vi "Measure vs B2Dv8.vi"() -> ()   [LabVIEW 2009]
doc: "This VI is an example operator panel.\n\nThe VI contains a table for the field values that may be configured manually, or loaded by checking the \"Prompt for File\" box. The data file should contain 3 columns of data, with each column delimited by a tab character.\n\nBefore the VI is executed, set the desired field units and coordinate system. Once the VI is started, follow the directions in the STATUS indicator to operate. Once a field value is achieved, it will be held indefinitely with no user intervention.\n\nThe present field is displayed in the selected units and coordinate system. The present field is queried once per second.\n\nIf a field point is specified that is outside the limits for the magnet, the VI will abort execution."
uses:
  <vilib>/Utility/file.llb/Read From Spreadsheet File (DBL).vi
panel:
  in  "Nr. of Accumulations":i32=5
  out "appended array":dbl[](array[numeric])=[3.4997816518320115, 222.76394903933627, 0.0, 0.0, 0.0, 0.0, 0.0, 0.0, 0.0, 0.0, 26.935568000000004, 3405678871.716173]
  in  "X Axis":enum16{"B", "phi"}(ring)=enum."phi"
  in  "Y Axis":T1(ring)=enum."HP (V)"
  out "XY Graph":T2(graph)
  in  "GPIB HP 2":string="13"
  in  "Wait between \nVectors":bool=TRUE
  in  "Change\nPID\n(polar coordinates)":bool=TRUE
  in  "Wait between \nVectors (ms)":u32=4000
  out "measured data":dbl[][](array[numeric])=[[3.500030260354902, 90.02209961014816, 0.0, 0.0, 0.0, 0.0, 0.0, 0.0, 0.0, 0.0, -94.19115, 3405672865.0000706], [3.5000353306931054, 90.40008745596127, 0.0, 0.0, 0.0, 0.0, 0.0, 0.0, 0.0, 0.0, -93.17439999999999, 3405672888.556781], [3.500010167370946, 90.77498772333144, 0.0, 0.0, 0.0, 0.0, 0.0, 0.0, 0.0, 0.0, -92.12794, 3405672906.302329], [3.499961687061731, 91.1795707814255, 0.0, 0.0, 0.0, 0.0, 0.0, 0.0, 0.0, 0.0, -90.85747400000001, 3405672924.971062], [3.50004724865251, 91.57794022797674, 0.0, 0.0, 0.0, 0.0, 0.0, 0.0, 0.0, 0.0, -88.536796, 3405672943.172702], [3.500004245611711, 91.97742193199196, 0.0, 0.0, 0.0, 0.0, 0.0, 0.0, 0.0, 0.0, -86.630854, 3405672961.1512966], [3.499981515165474, 92.3769958711717, 0.0, 0.0, 0.0, 0.0, 0.0, 0.0, 0.0, 0.0, -84.437106, 3405672979.515969], [3.499989652556133, 92.77683009737729, 0.0, 0.0, 0.0, 0.0, 0.0, 0.0, 0.0, 0.0, -82.45712800000001, 3405672997.6575966], [3.499997929856531, 93.17958494444387, 0.0, 0.0, 0.0, 0.0, 0.0, 0.0, 0.0, 0.0, -80.15669, 3405673015.994263], [3.4999788975649553, 93.57973481313714, 0.0, 0.0, 0.0, 0.0, 0.0, 0.0, 0.0, 0.0, -77.925174, 3405673034.877039], [3.50003012194181, 93.97981982914929, 0.0, 0.0, 0.0, 0.0, 0.0, 0.0, 0.0, 0.0, -75.205726, 3405673052.8976426], [3.4999928001068805, 94.37806425473491, 0.0, 0.0, 0.0, 0.0, 0.0, 0.0, 0.0, 0.0, -72.669112, 3405673070.9132447], [3.5000066802793395, 94.77875900181826, 0.0, 0.0, 0.0, 0.0, 0.0, 0.0, 0.0, 0.0, -69.859166, 3405673089.0468707], [3.499968184726827, 95.17532458941045, 0.0, 0.0, 0.0, 0.0, 0.0, 0.0, 0.0, 0.0, -66.825818, 3405673107.0374684], [3.499973556528678, 95.57470930884492, 0.0, 0.0, 0.0, 0.0, 0.0, 0.0, 0.0, 0.0, -63.7532, 3405673125.491158], [3.4999261373920447, 95.97066938046576, 0.0, 0.0, 0.0, 0.0, 0.0, 0.0, 0.0, 0.0, -60.45445599999999, 3405673143.7017994], [3.5000298004588473, 96.38048701574986, 0.0, 0.0, 0.0, 0.0, 0.0, 0.0, 0.0, 0.0, -57.068999999999996, 3405673162.2455077], [3.500064831970974, 96.77557569619363, 0.0, 0.0, 0.0, 0.0, 0.0, 0.0, 0.0, 0.0, -53.408407999999994, 3405673180.1530886], [3.4999764736352157, 97.1788243385936, 0.0, 0.0, 0.0, 0.0, 0.0, 0.0, 0.0, 0.0, -49.82861199999999, 3405673198.7077985], [3.499899112903114, 97.5720228055998, 0.0, 0.0, 0.0, 0.0, 0.0, 0.0, 0.0, 0.0, -46.072646, 3405673217.375531], [3.4999856331847994, 97.97927285454584, 0.0, 0.0, 0.0, 0.0, 0.0, 0.0, 0.0, 0.0, -42.447092, 3405673235.5991755], [3.4999729959101114, 98.3805293531586, 0.0, 0.0, 0.0, 0.0, 0.0, 0.0, 0.0, 0.0, -38.347238, 3405673254.280911], [3.499991174417444, 98.77649336396482, 0.0, 0.0, 0.0, 0.0, 0.0, 0.0, 0.0, 0.0, -34.288334, 3405673272.973649], [3.5000539345844377, 99.1754114769969, 0.0, 0.0, 0.0, 0.0, 0.0, 0.0, 0.0, 0.0, -30.040484, 3405673291.4163365], [3.5000102512135594, 99.57505833083601, 0.0, 0.0, 0.0, 0.0, 0.0, 0.0, 0.0, 0.0, -25.978331999999998, 3405673309.6199765], [3.5000214011488553, 99.98001455890109, 0.0, 0.0, 0.0, 0.0, 0.0, 0.0, 0.0, 0.0, -21.579306000000003, 3405673327.64058], [3.4999851274255445, 100.3796233603908, 0.0, 0.0, 0.0, 0.0, 0.0, 0.0, 0.0, 0.0, -17.288418, 3405673346.434338], [3.499954446117835, 100.77906761278494, 0.0, 0.0, 0.0, 0.0, 0.0, 0.0, 0.0, 0.0, -12.950921999999998, 3405673365.5421586], [3.4999038351503318, 101.17711177650253, 0.0, 0.0, 0.0, 0.0, 0.0, 0.0, 0.0, 0.0, -8.468328, 3405673383.8398175], [3.5000326492762897, 101.57761950670657, 0.0, 0.0, 0.0, 0.0, 0.0, 0.0, 0.0, 0.0, -4.102902, 3405673402.066462], [3.5000535285620993, 101.98021835524455, 0.0, 0.0, 0.0, 0.0, 0.0, 0.0, 0.0, 0.0, 0.38745399999999997, 3405673420.2901063], [3.4999165652340913, 102.3749303639201, 0.0, 0.0, 0.0, 0.0, 0.0, 0.0, 0.0, 0.0, 4.841813999999999, 3405673438.627773], [3.5000474151074012, 102.77699848468114, 0.0, 0.0, 0.0, 0.0, 0.0, 0.0, 0.0, 0.0, 9.427456000000001, 3405673456.962439], [3.4999308826603994, 103.17911248439914, 0.0, 0.0, 0.0, 0.0, 0.0, 0.0, 0.0, 0.0, 13.765427999999998, 3405673475.7191896], [3.5000704905187265, 103.57366085912142, 0.0, 0.0, 0.0, 0.0, 0.0, 0.0, 0.0, 0.0, 261.09814400000005, 3405673493.5167484], [3.4999923875488643, 103.97478211562277, 0.0, 0.0, 0.0, 0.0, 0.0, 0.0, 0.0, 0.0, 265.36180399999995, 3405673511.973439], [3.50008904903861, 104.37808498401525, 0.0, 0.0, 0.0, 0.0, 0.0, 0.0, 0.0, 0.0, 229.417352, 3405673530.1890817], [3.4999492656037177, 104.77837537502313, 0.0, 0.0, 0.0, 0.0, 0.0, 0.0, 0.0, 0.0, 232.49712, 3405673548.7317896], [3.50001056744119, 105.17362498473213, 0.0, 0.0, 0.0, 0.0, 0.0, 0.0, 0.0, 0.0, 235.83822400000003, 3405673567.045451], [3.5000558796967804, 105.57885121352332, 0.0, 0.0, 0.0, 0.0, 0.0, 0.0, 0.0, 0.0, 239.56730199999998, 3405673585.022046], [3.5000177358693487, 105.97640425681314, 0.0, 0.0, 0.0, 0.0, 0.0, 0.0, 0.0, 0.0, 243.122376, 3405673602.891619], [3.4999674469914717, 106.37839889947139, 0.0, 0.0, 0.0, 0.0, 0.0, 0.0, 0.0, 0.0, 246.787238, 3405673621.187278], [3.500025662334492, 106.77351906308944, 0.0, 0.0, 0.0, 0.0, 0.0, 0.0, 0.0, 0.0, 250.36398, 3405673639.0798554], [3.4999864297022643, 107.1790231276539, 0.0, 0.0, 0.0, 0.0, 0.0, 0.0, 0.0, 0.0, 254.03527200000002, 3405673657.559551], [3.499721066628025, 107.56702129634458, 0.0, 0.0, 0.0, 0.0, 0.0, 0.0, 0.0, 0.0, 257.475188, 3405673675.4481277], [3.500111289673516, 107.97687064757908, 0.0, 0.0, 0.0, 0.0, 0.0, 0.0, 0.0, 0.0, 261.015894, 3405673693.4397254], [3.499884412377072, 108.3738615102185, 0.0, 0.0, 0.0, 0.0, 0.0, 0.0, 0.0, 0.0, 264.300374, 3405673711.7653894], [3.5000656501557232, 108.77888564489481, 0.0, 0.0, 0.0, 0.0, 0.0, 0.0, 0.0, 0.0, 266.99548200000004, 3405673729.8580074], [3.500043560086075, 109.17352257915907, 0.0, 0.0, 0.0, 0.0, 0.0, 0.0, 0.0, 0.0, 267.42818, 3405673747.57455], [3.5001776575625416, 109.57306756392474, 0.0, 0.0, 0.0, 0.0, 0.0, 0.0, 0.0, 0.0, 267.436332, 3405673765.494133], [3.5000026075561714, 109.97733029781173, 0.0, 0.0, 0.0, 0.0, 0.0, 0.0, 0.0, 0.0, 267.448376, 3405673783.7847905], [3.5001300911251856, 110.3778645180017, 0.0, 0.0, 0.0, 0.0, 0.0, 0.0, 0.0, 0.0, 267.439162, 3405673801.9984326], [3.4999804328738757, 110.77378002437662, 0.0, 0.0, 0.0, 0.0, 0.0, 0.0, 0.0, 0.0, 267.450232, 3405673819.8710065], [3.499876745744056, 111.17592095148544, 0.0, 0.0, 0.0, 0.0, 0.0, 0.0, 0.0, 0.0, 267.40882, 3405673838.231678], [3.4999703288170885, 111.57508835663016, 0.0, 0.0, 0.0, 0.0, 0.0, 0.0, 0.0, 0.0, 267.457796, 3405673856.4593225], [3.500119241540208, 111.97744287188773, 0.0, 0.0, 0.0, 0.0, 0.0, 0.0, 0.0, 0.0, 267.418864, 3405673874.6969695], [3.49972657653423, 112.37499691140242, 0.0, 0.0, 0.0, 0.0, 0.0, 0.0, 0.0, 0.0, 267.38881, 3405673893.163662], [3.4999270649686403, 112.77733737785826, 0.0, 0.0, 0.0, 0.0, 0.0, 0.0, 0.0, 0.0, 267.381224, 3405673911.9984283], [3.5000914626335127, 113.1741296651589, 0.0, 0.0, 0.0, 0.0, 0.0, 0.0, 0.0, 0.0, 267.36403, 3405673929.7489777], [3.4998622755188524, 113.57559010596982, 0.0, 0.0, 0.0, 0.0, 0.0, 0.0, 0.0, 0.0, 267.36007, 3405673948.172662], [3.5001490743824046, 113.97242817412064, 0.0, 0.0, 0.0, 0.0, 0.0, 0.0, 0.0, 0.0, 267.321324, 3405673965.798186], [3.4999802161869433, 114.37362621591762, 0.0, 0.0, 0.0, 0.0, 0.0, 0.0, 0.0, 0.0, 267.356902, 3405673983.646755], [3.5000563137183955, 114.77392864162485, 0.0, 0.0, 0.0, 0.0, 0.0, 0.0, 0.0, 0.0, 267.323764, 3405674001.500325], [3.49993119076647, 115.17470533827793, 0.0, 0.0, 0.0, 0.0, 0.0, 0.0, 0.0, 0.0, 267.308444, 3405674019.6929626], [3.5000648210140337, 115.57734630667247, 0.0, 0.0, 0.0, 0.0, 0.0, 0.0, 0.0, 0.0, 267.31886399999996, 3405674038.1306496], [3.500079900873693, 115.97388455106301, 0.0, 0.0, 0.0, 0.0, 0.0, 0.0, 0.0, 0.0, 267.396796, 3405674056.340291], [3.500083588273286, 116.37112251486363, 0.0, 0.0, 0.0, 0.0, 0.0, 0.0, 0.0, 0.0, 267.36528, 3405674074.555933], [3.4998901857201177, 116.77465805491228, 0.0, 0.0, 0.0, 0.0, 0.0, 0.0, 0.0, 0.0, 267.285414, 3405674092.4365087], [3.4999827229287863, 117.1721217046015, 0.0, 0.0, 0.0, 0.0, 0.0, 0.0, 0.0, 0.0, 267.283164, 3405674110.184057], [3.4999878866361804, 117.57708722062549, 0.0, 0.0, 0.0, 0.0, 0.0, 0.0, 0.0, 0.0, 267.273348, 3405674128.629746], [3.5001579615211655, 117.97544473706006, 0.0, 0.0, 0.0, 0.0, 0.0, 0.0, 0.0, 0.0, 267.252734, 3405674146.844388], [3.4999645343488845, 118.7745823253807, 0.0, 0.0, 0.0, 0.0, 0.0, 0.0, 0.0, 0.0, 116.65878799999999, 3405674205.3390846], [3.5001504496235594, 119.17108378767131, 0.0, 0.0, 0.0, 0.0, 0.0, 0.0, 0.0, 0.0, 121.30668800000001, 3405674223.479712], [3.4998711554141537, 119.5754721818303, 0.0, 0.0, 0.0, 0.0, 0.0, 0.0, 0.0, 0.0, 125.380242, 3405674241.4823117], [3.499923475520572, 119.97879792281874, 0.0, 0.0, 0.0, 0.0, 0.0, 0.0, 0.0, 0.0, 129.742514, 3405674259.72596], [3.5001310719743053, 120.37543480515174, 0.0, 0.0, 0.0, 0.0, 0.0, 0.0, 0.0, 0.0, 133.87113399999998, 3405674277.4935126], [3.4999267634194866, 120.77174927933098, 0.0, 0.0, 0.0, 0.0, 0.0, 0.0, 0.0, 0.0, 138.492662, 3405674296.1472425], [3.49991499658206, 121.18047092404115, 0.0, 0.0, 0.0, 0.0, 0.0, 0.0, 0.0, 0.0, 141.84497799999997, 3405674314.1458416], [3.4999187174133057, 121.57140277391103, 0.0, 0.0, 0.0, 0.0, 0.0, 0.0, 0.0, 0.0, 142.904816, 3405674332.0884295], [3.4999151814008296, 121.97794839560709, 0.0, 0.0, 0.0, 0.0, 0.0, 0.0, 0.0, 0.0, 143.102296, 3405674350.8281765], [3.4999743592775077, 122.3763481541459, 0.0, 0.0, 0.0, 0.0, 0.0, 0.0, 0.0, 0.0, 142.739766, 3405674369.264863], [3.499865045655332, 122.77399110512413, 0.0, 0.0, 0.0, 0.0, 0.0, 0.0, 0.0, 0.0, 142.243708, 3405674387.8955884], [3.4998203203307456, 123.17412172298447, 0.0, 0.0, 0.0, 0.0, 0.0, 0.0, 0.0, 0.0, 141.711882, 3405674405.8771844], [3.5000601994965743, 123.57261234589748, 0.0, 0.0, 0.0, 0.0, 0.0, 0.0, 0.0, 0.0, 141.070174, 3405674424.2158513], [3.4998794808535916, 123.97398235246743, 0.0, 0.0, 0.0, 0.0, 0.0, 0.0, 0.0, 0.0, 140.32428, 3405674442.282464], [3.4998183876452793, 124.37992516662331, 0.0, 0.0, 0.0, 0.0, 0.0, 0.0, 0.0, 0.0, 139.541306, 3405674461.3902845], [3.4996747117553655, 124.76886652695832, 0.0, 0.0, 0.0, 0.0, 0.0, 0.0, 0.0, 0.0, 138.643932, 3405674479.8029666], [3.499920492725513, 125.17761969278995, 0.0, 0.0, 0.0, 0.0, 0.0, 0.0, 0.0, 0.0, 137.71333600000003, 3405674498.320669], [3.499892731684787, 125.57286533774852, 0.0, 0.0, 0.0, 0.0, 0.0, 0.0, 0.0, 0.0, 136.705396, 3405674516.3372717], [3.4998363633175766, 125.97345124665485, 0.0, 0.0, 0.0, 0.0, 0.0, 0.0, 0.0, 0.0, 135.692706, 3405674534.5299096], [3.499870126161827, 126.3758198674582, 0.0, 0.0, 0.0, 0.0, 0.0, 0.0, 0.0, 0.0, 134.685222, 3405674552.6985426], [3.4997484133720245, 126.7789053690341, 0.0, 0.0, 0.0, 0.0, 0.0, 0.0, 0.0, 0.0, 133.609004, 3405674571.6863394], [3.499957391926365, 127.17429070452764, 0.0, 0.0, 0.0, 0.0, 0.0, 0.0, 0.0, 0.0, 132.455004, 3405674589.79196], [3.499677578577775, 127.57042872059915, 0.0, 0.0, 0.0, 0.0, 0.0, 0.0, 0.0, 0.0, 131.30946, 3405674607.74755], [3.500054207151655, 127.97261410503376, 0.0, 0.0, 0.0, 0.0, 0.0, 0.0, 0.0, 0.0, 130.105918, 3405674625.7691536], [3.499849894738345, 128.37151254032418, 0.0, 0.0, 0.0, 0.0, 0.0, 0.0, 0.0, 0.0, 128.936262, 3405674643.644728], [3.4997748452436195, 128.77222922792825, 0.0, 0.0, 0.0, 0.0, 0.0, 0.0, 0.0, 0.0, 127.730572, 3405674661.544307], [3.4999212348994373, 129.1762854888641, 0.0, 0.0, 0.0, 0.0, 0.0, 0.0, 0.0, 0.0, 126.478984, 3405674679.989996], [3.4998989024541842, 129.56836012091844, 0.0, 0.0, 0.0, 0.0, 0.0, 0.0, 0.0, 0.0, 125.223346, 3405674698.1766324], [3.4998525424508964, 129.97688401087316, 0.0, 0.0, 0.0, 0.0, 0.0, 0.0, 0.0, 0.0, 124.11873599999998, 3405674716.1652293], [3.4999583698667047, 130.37049879363013, 0.0, 0.0, 0.0, 0.0, 0.0, 0.0, 0.0, 0.0, 122.84383, 3405674734.031802], [3.5000659052223577, 130.77199786281247, 0.0, 0.0, 0.0, 0.0, 0.0, 0.0, 0.0, 0.0, 121.54545200000001, 3405674752.1194186], [3.499940835514223, 131.17010929315063, 0.0, 0.0, 0.0, 0.0, 0.0, 0.0, 0.0, 0.0, 120.19422200000001, 3405674769.889972], [3.4997394238571538, 131.57332378320737, 0.0, 0.0, 0.0, 0.0, 0.0, 0.0, 0.0, 0.0, 118.95105799999999, 3405674788.121618], [3.4997819649943906, 131.97662577132326, 0.0, 0.0, 0.0, 0.0, 0.0, 0.0, 0.0, 0.0, 117.512268, 3405674806.726338], [3.499631089414997, 132.37185861748466, 0.0, 0.0, 0.0, 0.0, 0.0, 0.0, 0.0, 0.0, 116.241782, 3405674825.1970315], [3.4999101294890416, 132.775384040791, 0.0, 0.0, 0.0, 0.0, 0.0, 0.0, 0.0, 0.0, 114.91744399999999, 3405674842.9615836], [3.4999685907733515, 133.17051292372958, 0.0, 0.0, 0.0, 0.0, 0.0, 0.0, 0.0, 0.0, 114.30012199999999, 3405674861.3792663], [3.4996256947565123, 133.5715146285057, 0.0, 0.0, 0.0, 0.0, 0.0, 0.0, 0.0, 0.0, 112.842244, 3405674879.8129525], [3.5001002197365723, 133.9639663607044, 0.0, 0.0, 0.0, 0.0, 0.0, 0.0, 0.0, 0.0, 111.453706, 3405674897.649519], [3.4997285691893314, 134.3653691446759, 0.0, 0.0, 0.0, 0.0, 0.0, 0.0, 0.0, 0.0, 110.01489600000001, 3405674915.6151114], [3.5001733746344623, 134.76213466710348, 0.0, 0.0, 0.0, 0.0, 0.0, 0.0, 0.0, 0.0, 108.53296399999999, 3405674933.137615], [3.499762188563674, 135.16750903999028, 0.0, 0.0, 0.0, 0.0, 0.0, 0.0, 0.0, 0.0, 107.14234200000001, 3405674951.1822233], [3.499836914614737, 135.5722129165841, 0.0, 0.0, 0.0, 0.0, 0.0, 0.0, 0.0, 0.0, 105.73913399999999, 3405674969.165819], [3.4995520173016432, 135.97320750746104, 0.0, 0.0, 0.0, 0.0, 0.0, 0.0, 0.0, 0.0, 104.295556, 3405674987.727531], [3.4997063943708193, 136.3784270813745, 0.0, 0.0, 0.0, 0.0, 0.0, 0.0, 0.0, 0.0, 102.898618, 3405675005.963177], [3.4997487944708263, 136.77400815747285, 0.0, 0.0, 0.0, 0.0, 0.0, 0.0, 0.0, 0.0, 101.375878, 3405675024.188822], [3.499675371516622, 137.1697360955709, 0.0, 0.0, 0.0, 0.0, 0.0, 0.0, 0.0, 0.0, 99.769748, 3405675042.1754184], [3.5000946885762967, 137.56035636171558, 0.0, 0.0, 0.0, 0.0, 0.0, 0.0, 0.0, 0.0, 98.309808, 3405675060.0249877], [3.5000500578134592, 137.96321622018945, 0.0, 0.0, 0.0, 0.0, 0.0, 0.0, 0.0, 0.0, 96.905448, 3405675077.7435308], [3.4998388080738803, 138.36813289223542, 0.0, 0.0, 0.0, 0.0, 0.0, 0.0, 0.0, 0.0, 95.43121000000001, 3405675095.999181], [3.500244357712759, 138.75786944236057, 0.0, 0.0, 0.0, 0.0, 0.0, 0.0, 0.0, 0.0, 93.957746, 3405675113.292639], [3.500018961548637, 139.16851720473673, 0.0, 0.0, 0.0, 0.0, 0.0, 0.0, 0.0, 0.0, 92.531196, 3405675131.40326], [3.499807575924711, 139.57430436350464, 0.0, 0.0, 0.0, 0.0, 0.0, 0.0, 0.0, 0.0, 91.072, 3405675149.1228037], [3.4996448960716005, 139.9696103533873, 0.0, 0.0, 0.0, 0.0, 0.0, 0.0, 0.0, 0.0, 89.58736, 3405675167.702519], [3.4998269038625325, 140.3724506193979, 0.0, 0.0, 0.0, 0.0, 0.0, 0.0, 0.0, 0.0, 88.050864, 3405675185.6941166], [3.4996307826540787, 140.77230184499527, 0.0, 0.0, 0.0, 0.0, 0.0, 0.0, 0.0, 0.0, 86.52822800000001, 3405675203.7967362], [3.4999209362498465, 141.16183906424567, 0.0, 0.0, 0.0, 0.0, 0.0, 0.0, 0.0, 0.0, 84.84612999999999, 3405675221.6573076], [3.4998077249043273, 141.57216537456776, 0.0, 0.0, 0.0, 0.0, 0.0, 0.0, 0.0, 0.0, 83.383914, 3405675239.980972], [3.499697436993662, 141.973171053346, 0.0, 0.0, 0.0, 0.0, 0.0, 0.0, 0.0, 0.0, 81.705942, 3405675258.216618], [3.4998543302971914, 142.36464159300596, 0.0, 0.0, 0.0, 0.0, 0.0, 0.0, 0.0, 0.0, 80.12457, 3405675275.940162], [3.4999124462477633, 142.76657365570128, 0.0, 0.0, 0.0, 0.0, 0.0, 0.0, 0.0, 0.0, 78.74135, 3405675293.802734], [3.499690775625755, 143.16824834609835, 0.0, 0.0, 0.0, 0.0, 0.0, 0.0, 0.0, 0.0, 77.283612, 3405675311.322237], [3.4997128073314814, 143.56064585097945, 0.0, 0.0, 0.0, 0.0, 0.0, 0.0, 0.0, 0.0, 75.68050799999999, 3405675328.8597436], [3.5001708675148993, 143.96192746465903, 0.0, 0.0, 0.0, 0.0, 0.0, 0.0, 0.0, 0.0, 74.109934, 3405675346.636298], [3.499657025781241, 144.3712166445686, 0.0, 0.0, 0.0, 0.0, 0.0, 0.0, 0.0, 0.0, 72.44393400000001, 3405675364.734917], [3.4995117024522155, 144.77137592091586, 0.0, 0.0, 0.0, 0.0, 0.0, 0.0, 0.0, 0.0, 70.77924, 3405675382.80353], [3.499820175166147, 145.16460180655824, 0.0, 0.0, 0.0, 0.0, 0.0, 0.0, 0.0, 0.0, 68.983552, 3405675400.820133], [3.500028838695476, 145.55913599705326, 0.0, 0.0, 0.0, 0.0, 0.0, 0.0, 0.0, 0.0, 67.301224, 3405675418.6897063], [3.499829354482873, 145.96839372143788, 0.0, 0.0, 0.0, 0.0, 0.0, 0.0, 0.0, 0.0, 65.67662800000001, 3405675436.2842245], [3.499874279184897, 146.36659724897362, 0.0, 0.0, 0.0, 0.0, 0.0, 0.0, 0.0, 0.0, 63.974917999999995, 3405675453.929753], [3.499740963971477, 146.76926640518522, 0.0, 0.0, 0.0, 0.0, 0.0, 0.0, 0.0, 0.0, 62.24362, 3405675471.798326], [3.499957562899871, 147.16232155540825, 0.0, 0.0, 0.0, 0.0, 0.0, 0.0, 0.0, 0.0, 60.423671999999996, 3405675489.1938043], [3.499774684533277, 147.56495699983415, 0.0, 0.0, 0.0, 0.0, 0.0, 0.0, 0.0, 0.0, 58.586968000000006, 3405675507.045374], [3.4997879960077585, 147.96669508570739, 0.0, 0.0, 0.0, 0.0, 0.0, 0.0, 0.0, 0.0, 56.697368, 3405675524.6008844], [3.5003051893513515, 148.35772126463573, 0.0, 0.0, 0.0, 0.0, 0.0, 0.0, 0.0, 0.0, 54.69736399999999, 3405675542.7595153], [3.5000712640316345, 148.76002104541612, 0.0, 0.0, 0.0, 0.0, 0.0, 0.0, 0.0, 0.0, 52.805948, 3405675560.174998], [3.4998644637328464, 149.16474645537087, 0.0, 0.0, 0.0, 0.0, 0.0, 0.0, 0.0, 0.0, 50.935509999999994, 3405675578.1235867], [3.4999181319710893, 149.55741350777478, 0.0, 0.0, 0.0, 0.0, 0.0, 0.0, 0.0, 0.0, 48.771522, 3405675595.9831576], [3.499928801690115, 149.96245893805968, 0.0, 0.0, 0.0, 0.0, 0.0, 0.0, 0.0, 0.0, 46.733486, 3405675613.827726], [3.499850763246913, 150.36182484047603, 0.0, 0.0, 0.0, 0.0, 0.0, 0.0, 0.0, 0.0, 44.20468, 3405675631.804321], [3.499757492812895, 150.76493211594644, 0.0, 0.0, 0.0, 0.0, 0.0, 0.0, 0.0, 0.0, 41.787772, 3405675650.024964], [3.5000510570561683, 151.159314109217, 0.0, 0.0, 0.0, 0.0, 0.0, 0.0, 0.0, 0.0, 39.269336, 3405675667.7705126], [3.5000198440866015, 151.55950038401437, 0.0, 0.0, 0.0, 0.0, 0.0, 0.0, 0.0, 0.0, 36.84650799999999, 3405675685.822122], [3.499885385551933, 151.96322058038277, 0.0, 0.0, 0.0, 0.0, 0.0, 0.0, 0.0, 0.0, 34.164786, 3405675703.46565], [3.500161274012956, 152.35955557611751, 0.0, 0.0, 0.0, 0.0, 0.0, 0.0, 0.0, 0.0, 31.506318, 3405675721.31922], [3.499590042747865, 152.76732800027264, 0.0, 0.0, 0.0, 0.0, 0.0, 0.0, 0.0, 0.0, 29.173270000000002, 3405675738.9447446], [3.499970654919838, 153.15667471181055, 0.0, 0.0, 0.0, 0.0, 0.0, 0.0, 0.0, 0.0, 26.248548, 3405675756.4292407], [3.499702667441907, 153.57405951439412, 0.0, 0.0, 0.0, 0.0, 0.0, 0.0, 0.0, 0.0, 23.492397999999998, 3405675774.368828], [3.5001161369588867, 153.95919456149448, 0.0, 0.0, 0.0, 0.0, 0.0, 0.0, 0.0, 0.0, 20.466725999999998, 3405675791.98235], [3.499761557363587, 154.36218214966078, 0.0, 0.0, 0.0, 0.0, 0.0, 0.0, 0.0, 0.0, 17.731626, 3405675809.865926], [3.499855255578436, 154.76681122212005, 0.0, 0.0, 0.0, 0.0, 0.0, 0.0, 0.0, 0.0, 14.674454, 3405675827.5584636], [3.499861412641935, 155.1627389738173, 0.0, 0.0, 0.0, 0.0, 0.0, 0.0, 0.0, 0.0, 11.691854, 3405675845.3200154], [3.4996201464301806, 155.56922894473985, 0.0, 0.0, 0.0, 0.0, 0.0, 0.0, 0.0, 0.0, 8.983192, 3405675863.3246155], [3.500049102984128, 155.95480385736514, 0.0, 0.0, 0.0, 0.0, 0.0, 0.0, 0.0, 0.0, 5.7563, 3405675881.00215], [3.499825275481621, 156.36161382626045, 0.0, 0.0, 0.0, 0.0, 0.0, 0.0, 0.0, 0.0, 3.06459, 3405675899.062762], [3.499755668185996, 156.76598299473588, 0.0, 0.0, 0.0, 0.0, 0.0, 0.0, 0.0, 0.0, 0.370134, 3405675916.5812645], [3.4999229571091988, 157.16243095877633, 0.0, 0.0, 0.0, 0.0, 0.0, 0.0, 0.0, 0.0, -2.491728, 3405675934.541856], [3.499652875143477, 157.56907909621776, 0.0, 0.0, 0.0, 0.0, 0.0, 0.0, 0.0, 0.0, -4.861262, 3405675952.6384745], [3.499898464270071, 157.9624759786651, 0.0, 0.0, 0.0, 0.0, 0.0, 0.0, 0.0, 0.0, -7.467224, 3405675970.4420347], [3.4999046228433137, 158.35827965552573, 0.0, 0.0, 0.0, 0.0, 0.0, 0.0, 0.0, 0.0, -10.00578, 3405675987.738493], [3.4999049466235514, 158.7631499898759, 0.0, 0.0, 0.0, 0.0, 0.0, 0.0, 0.0, 0.0, -12.342396, 3405676005.1589766], [3.499848603154142, 159.1669087738777, 0.0, 0.0, 0.0, 0.0, 0.0, 0.0, 0.0, 0.0, -14.602238000000002, 3405676022.684481], [3.499799771144058, 159.56999589162385, 0.0, 0.0, 0.0, 0.0, 0.0, 0.0, 0.0, 0.0, -16.682208, 3405676040.5450525], [3.5001060343081036, 159.9591748912087, 0.0, 0.0, 0.0, 0.0, 0.0, 0.0, 0.0, 0.0, -18.971415999999998, 3405676058.2735972], [3.499963705526102, 160.3577384555535, 0.0, 0.0, 0.0, 0.0, 0.0, 0.0, 0.0, 0.0, -21.064362000000003, 3405676075.99014], [3.4999610849979463, 160.75770616282318, 0.0, 0.0, 0.0, 0.0, 0.0, 0.0, 0.0, 0.0, -23.199610000000003, 3405676093.2665944], [3.4999863803306432, 161.15841490681555, 0.0, 0.0, 0.0, 0.0, 0.0, 0.0, 0.0, 0.0, -25.005322, 3405676111.017144], [3.4997685832351837, 161.56701846035787, 0.0, 0.0, 0.0, 0.0, 0.0, 0.0, 0.0, 0.0, -26.69855, 3405676128.885717], [3.499864297212108, 161.96724937012618, 0.0, 0.0, 0.0, 0.0, 0.0, 0.0, 0.0, 0.0, -28.503346, 3405676146.6412673], [3.499987715535585, 162.35913630673681, 0.0, 0.0, 0.0, 0.0, 0.0, 0.0, 0.0, 0.0, -30.283129999999996, 3405676164.2857957], [3.499811491437789, 162.76713470966794, 0.0, 0.0, 0.0, 0.0, 0.0, 0.0, 0.0, 0.0, -31.94392, 3405676181.936325], [3.4997372896261805, 163.17358269779734, 0.0, 0.0, 0.0, 0.0, 0.0, 0.0, 0.0, 0.0, -33.542836, 3405676200.155968], [3.4997971091050406, 163.57368005360183, 0.0, 0.0, 0.0, 0.0, 0.0, 0.0, 0.0, 0.0, -35.172394, 3405676218.4176197], [3.499894991481888, 163.96647788399946, 0.0, 0.0, 0.0, 0.0, 0.0, 0.0, 0.0, 0.0, -37.037714, 3405676235.9141183], [3.499851909209874, 164.36191539785457, 0.0, 0.0, 0.0, 0.0, 0.0, 0.0, 0.0, 0.0, -38.72648, 3405676253.7726893], [3.500009697200852, 164.75342406619708, 0.0, 0.0, 0.0, 0.0, 0.0, 0.0, 0.0, 0.0, -40.503516, 3405676271.28019], [3.499658589134089, 165.1736317476941, 0.0, 0.0, 0.0, 0.0, 0.0, 0.0, 0.0, 0.0, -41.745548, 3405676289.28179], [3.499983900491544, 165.5628242409946, 0.0, 0.0, 0.0, 0.0, 0.0, 0.0, 0.0, 0.0, -43.531876, 3405676306.78529], [3.500036513295255, 165.95335429157527, 0.0, 0.0, 0.0, 0.0, 0.0, 0.0, 0.0, 0.0, -45.166786, 3405676324.195771], [3.4998375530587134, 166.3627599734219, 0.0, 0.0, 0.0, 0.0, 0.0, 0.0, 0.0, 0.0, -46.52648, 3405676341.929317], [3.500049134697969, 166.75391226698494, 0.0, 0.0, 0.0, 0.0, 0.0, 0.0, 0.0, 0.0, -48.326818, 3405676359.380807], [3.500087796570252, 167.16691392910417, 0.0, 0.0, 0.0, 0.0, 0.0, 0.0, 0.0, 0.0, -49.999303999999995, 3405676377.4424186], [3.500032535877345, 167.5562605251271, 0.0, 0.0, 0.0, 0.0, 0.0, 0.0, 0.0, 0.0, -52.00913200000001, 3405676395.594048], [3.5000170391013814, 167.95337755878842, 0.0, 0.0, 0.0, 0.0, 0.0, 0.0, 0.0, 0.0, -53.895382, 3405676413.111551], [3.4999200735588243, 168.3630082308151, 0.0, 0.0, 0.0, 0.0, 0.0, 0.0, 0.0, 0.0, -55.631879999999995, 3405676430.523032], [3.499955430987658, 168.7537960771341, 0.0, 0.0, 0.0, 0.0, 0.0, 0.0, 0.0, 0.0, -57.531048, 3405676448.0525374], [3.4997136615729008, 169.17084750147322, 0.0, 0.0, 0.0, 0.0, 0.0, 0.0, 0.0, 0.0, -58.97388, 3405676465.948116], [3.4998790576247063, 169.56729530466978, 0.0, 0.0, 0.0, 0.0, 0.0, 0.0, 0.0, 0.0, -60.83071799999999, 3405676483.8196898], [3.499857506270791, 169.96265958623903, 0.0, 0.0, 0.0, 0.0, 0.0, 0.0, 0.0, 0.0, -62.59072999999999, 3405676501.169159], [3.500079280530657, 170.35257762283075, 0.0, 0.0, 0.0, 0.0, 0.0, 0.0, 0.0, 0.0, -64.17150000000001, 3405676518.663657], [3.4998655609894507, 170.77400602981498, 0.0, 0.0, 0.0, 0.0, 0.0, 0.0, 0.0, 0.0, -65.488986, 3405676536.6252484], [3.5001123136265218, 171.15407335274932, 0.0, 0.0, 0.0, 0.0, 0.0, 0.0, 0.0, 0.0, -67.016374, 3405676554.247772], [3.4998982086055017, 171.5706378722838, 0.0, 0.0, 0.0, 0.0, 0.0, 0.0, 0.0, 0.0, -68.40785, 3405676571.993321], [3.4999106661884967, 171.96715748814316, 0.0, 0.0, 0.0, 0.0, 0.0, 0.0, 0.0, 0.0, -69.892408, 3405676589.7498713], [3.5000605179053697, 172.35995532473072, 0.0, 0.0, 0.0, 0.0, 0.0, 0.0, 0.0, 0.0, -71.53339, 3405676607.2923794], [3.5000721455707167, 172.76312695023654, 0.0, 0.0, 0.0, 0.0, 0.0, 0.0, 0.0, 0.0, -72.88933800000001, 3405676625.3529906], [3.4998116468461564, 173.17760321610658, 0.0, 0.0, 0.0, 0.0, 0.0, 0.0, 0.0, 0.0, -73.64847, 3405676643.3975987], [3.4997971071763576, 173.58004396801417, 0.0, 0.0, 0.0, 0.0, 0.0, 0.0, 0.0, 0.0, -74.254306, 3405676661.4902167], [3.5000250522817695, 173.95295844665097, 0.0, 0.0, 0.0, 0.0, 0.0, 0.0, 0.0, 0.0, -75.25022399999999, 3405676678.751668], [3.50000971662937, 174.35395992633687, 0.0, 0.0, 0.0, 0.0, 0.0, 0.0, 0.0, 0.0, -76.226776, 3405676696.4982166], [3.49987434010137, 174.77472768371223, 0.0, 0.0, 0.0, 0.0, 0.0, 0.0, 0.0, 0.0, -76.850642, 3405676714.731863], [3.4999964777839425, 175.15880027283484, 0.0, 0.0, 0.0, 0.0, 0.0, 0.0, 0.0, 0.0, -77.952372, 3405676732.2673693], [3.500049524292478, 175.55879525515346, 0.0, 0.0, 0.0, 0.0, 0.0, 0.0, 0.0, 0.0, -78.61368999999999, 3405676749.9108973], [3.4999613266434815, 175.9636495528889, 0.0, 0.0, 0.0, 0.0, 0.0, 0.0, 0.0, 0.0, -78.99387, 3405676767.894493], [3.4998957282324854, 176.37933633308913, 0.0, 0.0, 0.0, 0.0, 0.0, 0.0, 0.0, 0.0, -79.071402, 3405676785.9300995], [3.4999711401381584, 176.75808552799955, 0.0, 0.0, 0.0, 0.0, 0.0, 0.0, 0.0, 0.0, -79.425716, 3405676803.2145557], [3.4999191033508192, 177.186400055552, 0.0, 0.0, 0.0, 0.0, 0.0, 0.0, 0.0, 0.0, -79.268152, 3405676821.9012923], [3.500051738646159, 177.5529261960563, 0.0, 0.0, 0.0, 0.0, 0.0, 0.0, 0.0, 0.0, -79.56219200000001, 3405676839.4057927], [3.4999633862370616, 177.97144811675403, 0.0, 0.0, 0.0, 0.0, 0.0, 0.0, 0.0, 0.0, -78.995892, 3405676857.271365], [3.4999292172414003, 178.39727748214156, 0.0, 0.0, 0.0, 0.0, 0.0, 0.0, 0.0, 0.0, -78.078716, 3405676876.881286], [3.500050673490314, 178.75922180439102, 0.0, 0.0, 0.0, 0.0, 0.0, 0.0, 0.0, 0.0, -78.58030000000001, 3405676894.7508593], [3.499972748536766, 179.1865299705665, 0.0, 0.0, 0.0, 0.0, 0.0, 0.0, 0.0, 0.0, -77.18027599999999, 3405676914.092727], [3.499965262584759, 179.60006824213608, 0.0, 0.0, 0.0, 0.0, 0.0, 0.0, 0.0, 0.0, -74.848536, 3405676937.7784634], [3.4999900000142854, 179.9998362973051, 0.0, 0.0, 0.0, 0.0, 0.0, 0.0, 0.0, 0.0, -71.298726, 3405676966.0801225], [3.4999897106277333, 180.3616216837924, 0.0, 0.0, 0.0, 0.0, 0.0, 0.0, 0.0, 0.0, -70.349932, 3405676983.611628], [3.499979572997534, 180.76206078320823, 0.0, 0.0, 0.0, 0.0, 0.0, 0.0, 0.0, 0.0, -67.80041200000001, 3405677001.1971445], [3.500001028571278, 181.1630201450811, 0.0, 0.0, 0.0, 0.0, 0.0, 0.0, 0.0, 0.0, -64.201094, 3405677019.2797604], [3.500012225121507, 181.5809037716472, 0.0, 0.0, 0.0, 0.0, 0.0, 0.0, 0.0, 0.0, -58.284716, 3405677037.957495], [3.5000025518847835, 181.96710354335045, 0.0, 0.0, 0.0, 0.0, 0.0, 0.0, 0.0, 0.0, -53.596778, 3405677056.1591344], [3.500029927186338, 182.36844322666283, 0.0, 0.0, 0.0, 0.0, 0.0, 0.0, 0.0, 0.0, -50.810602, 3405677074.368776], [3.5000324859206664, 182.76761810743517, 0.0, 0.0, 0.0, 0.0, 0.0, 0.0, 0.0, 0.0, -49.464372, 3405677092.097321], [3.50004289185147, 183.17216621626477, 0.0, 0.0, 0.0, 0.0, 0.0, 0.0, 0.0, 0.0, 177.63958000000002, 3405677109.727846], [3.500017652098343, 183.56362116586928, 0.0, 0.0, 0.0, 0.0, 0.0, 0.0, 0.0, 0.0, 165.90623, 3405677127.15133], [3.500045806114543, 183.9622439038027, 0.0, 0.0, 0.0, 0.0, 0.0, 0.0, 0.0, 0.0, 162.92809, 3405677144.668833], [3.5000488600161, 184.375038778923, 0.0, 0.0, 0.0, 0.0, 0.0, 0.0, 0.0, 0.0, 161.92900600000002, 3405677162.836466], [3.5000339774636475, 184.75851652726013, 0.0, 0.0, 0.0, 0.0, 0.0, 0.0, 0.0, 0.0, 161.486364, 3405677180.492996], [3.4999905933730746, 185.15392326686992, 0.0, 0.0, 0.0, 0.0, 0.0, 0.0, 0.0, 0.0, 161.879634, 3405677198.1415253], [3.4999954614827717, 185.56151602721337, 0.0, 0.0, 0.0, 0.0, 0.0, 0.0, 0.0, 0.0, 162.130132, 3405677215.877072], [3.499980180515313, 185.95708014524186, 0.0, 0.0, 0.0, 0.0, 0.0, 0.0, 0.0, 0.0, 162.666296, 3405677233.5025964], [3.4999816312946557, 186.35866744347257, 0.0, 0.0, 0.0, 0.0, 0.0, 0.0, 0.0, 0.0, 163.14201400000002, 3405677251.335162], [3.5000057752095213, 186.75491948349216, 0.0, 0.0, 0.0, 0.0, 0.0, 0.0, 0.0, 0.0, 163.88484599999998, 3405677269.407776], [3.499993048907383, 187.16262084606458, 0.0, 0.0, 0.0, 0.0, 0.0, 0.0, 0.0, 0.0, 164.53717799999998, 3405677287.508395], [3.500029168164174, 187.5557214338629, 0.0, 0.0, 0.0, 0.0, 0.0, 0.0, 0.0, 0.0, 165.14878800000002, 3405677305.705034], [3.5000893729874956, 187.96779468380993, 0.0, 0.0, 0.0, 0.0, 0.0, 0.0, 0.0, 0.0, 166.213776, 3405677323.7066336], [3.5000398282591014, 188.3598507899822, 0.0, 0.0, 0.0, 0.0, 0.0, 0.0, 0.0, 0.0, 167.23951399999999, 3405677341.3451605], [3.5001832880579267, 188.7678919281932, 0.0, 0.0, 0.0, 0.0, 0.0, 0.0, 0.0, 0.0, 168.57080599999998, 3405677358.9726853], [3.499978074817041, 189.15538197853044, 0.0, 0.0, 0.0, 0.0, 0.0, 0.0, 0.0, 0.0, 169.872266, 3405677376.4541807], [3.499921177683863, 189.5575407517811, 0.0, 0.0, 0.0, 0.0, 0.0, 0.0, 0.0, 0.0, 171.32737400000002, 3405677394.313752], [3.500034605686064, 189.9557099300937, 0.0, 0.0, 0.0, 0.0, 0.0, 0.0, 0.0, 0.0, 172.72437200000002, 3405677411.8062496], [3.500025527735476, 190.35503879022, 0.0, 0.0, 0.0, 0.0, 0.0, 0.0, 0.0, 0.0, 174.599174, 3405677429.095707], [3.5000282847142823, 190.7565084167859, 0.0, 0.0, 0.0, 0.0, 0.0, 0.0, 0.0, 0.0, 176.47025000000002, 3405677446.694226], [3.4999545572621376, 191.15342008774758, 0.0, 0.0, 0.0, 0.0, 0.0, 0.0, 0.0, 0.0, 178.270402, 3405677464.5848036], [3.500067445435874, 191.56162887451444, 0.0, 0.0, 0.0, 0.0, 0.0, 0.0, 0.0, 0.0, 180.45824399999998, 3405677482.2343326], [3.500079063449853, 191.96640785272828, 0.0, 0.0, 0.0, 0.0, 0.0, 0.0, 0.0, 0.0, 182.564288, 3405677500.3189487], [3.499955161498501, 192.35870280441566, 0.0, 0.0, 0.0, 0.0, 0.0, 0.0, 0.0, 0.0, 184.53730000000002, 3405677518.050494], [3.500109684467046, 192.77038898399732, 0.0, 0.0, 0.0, 0.0, 0.0, 0.0, 0.0, 0.0, 186.670816, 3405677536.213126], [3.499920012243137, 193.15679331381895, 0.0, 0.0, 0.0, 0.0, 0.0, 0.0, 0.0, 0.0, 188.74021999999997, 3405677554.515786], [3.4999469379549177, 193.55410938685534, 0.0, 0.0, 0.0, 0.0, 0.0, 0.0, 0.0, 0.0, 190.92144000000002, 3405677572.0432906], [3.5001166463419473, 193.96668502332557, 0.0, 0.0, 0.0, 0.0, 0.0, 0.0, 0.0, 0.0, 193.381488, 3405677590.182918], [3.4999543991600803, 194.3609059522713, 0.0, 0.0, 0.0, 0.0, 0.0, 0.0, 0.0, 0.0, 195.711774, 3405677607.8544517], [3.4999559284368136, 194.7620939362642, 0.0, 0.0, 0.0, 0.0, 0.0, 0.0, 0.0, 0.0, 198.505814, 3405677625.391958], [3.499966958658324, 195.16160650126292, 0.0, 0.0, 0.0, 0.0, 0.0, 0.0, 0.0, 0.0, 201.037874, 3405677643.6956186], [3.5001020593405565, 195.55960798295925, 0.0, 0.0, 0.0, 0.0, 0.0, 0.0, 0.0, 0.0, 203.75619600000002, 3405677660.9850755], [3.500140975018007, 195.96084331908838, 0.0, 0.0, 0.0, 0.0, 0.0, 0.0, 0.0, 0.0, 206.448218, 3405677678.3725524], [3.5000045233827914, 196.36013501738597, 0.0, 0.0, 0.0, 0.0, 0.0, 0.0, 0.0, 0.0, 208.99730399999999, 3405677696.1020975], [3.5001622025271915, 196.76788736329806, 0.0, 0.0, 0.0, 0.0, 0.0, 0.0, 0.0, 0.0, 211.764756, 3405677714.209718], [3.500111751358805, 197.16348288627555, 0.0, 0.0, 0.0, 0.0, 0.0, 0.0, 0.0, 0.0, 214.02986800000002, 3405677732.1593075], [3.50013211556364, 197.56712323191735, 0.0, 0.0, 0.0, 0.0, 0.0, 0.0, 0.0, 0.0, 216.74170999999996, 3405677750.02388], [3.500096862102533, 197.96765415411394, 0.0, 0.0, 0.0, 0.0, 0.0, 0.0, 0.0, 0.0, 219.37103399999995, 3405677768.118498], [3.500109385162127, 198.36729120489656, 0.0, 0.0, 0.0, 0.0, 0.0, 0.0, 0.0, 0.0, 221.771094, 3405677786.0510836], [3.499889463468811, 198.7546229730515, 0.0, 0.0, 0.0, 0.0, 0.0, 0.0, 0.0, 0.0, 224.15211200000002, 3405677803.78563], [3.5000038445264603, 199.16317668561933, 0.0, 0.0, 0.0, 0.0, 0.0, 0.0, 0.0, 0.0, 226.482686, 3405677821.7472215], [3.499970860050124, 199.5615883845575, 0.0, 0.0, 0.0, 0.0, 0.0, 0.0, 0.0, 0.0, 228.8775, 3405677839.7098136], [3.50018806576161, 199.9708274515273, 0.0, 0.0, 0.0, 0.0, 0.0, 0.0, 0.0, 0.0, 231.317566, 3405677857.710413], [3.49988690773002, 200.35349898748, 0.0, 0.0, 0.0, 0.0, 0.0, 0.0, 0.0, 0.0, 233.27707400000003, 3405677875.410952], [3.5001638972196716, 200.76738862005774, 0.0, 0.0, 0.0, 0.0, 0.0, 0.0, 0.0, 0.0, 235.23017799999997, 3405677892.848439], [3.500268019523648, 201.16571626410652, 0.0, 0.0, 0.0, 0.0, 0.0, 0.0, 0.0, 0.0, 237.18301400000001, 3405677910.821033], [3.500113798107141, 201.55831793356268, 0.0, 0.0, 0.0, 0.0, 0.0, 0.0, 0.0, 0.0, 238.99041600000004, 3405677928.3135304], [3.499944680277104, 201.9563545042168, 0.0, 0.0, 0.0, 0.0, 0.0, 0.0, 0.0, 0.0, 240.75021399999997, 3405677945.824032], [3.5000955267678053, 202.36171270816067, 0.0, 0.0, 0.0, 0.0, 0.0, 0.0, 0.0, 0.0, 242.29263199999997, 3405677963.8996463], [3.4999853614836733, 202.76184588805626, 0.0, 0.0, 0.0, 0.0, 0.0, 0.0, 0.0, 0.0, 243.74934399999998, 3405677981.7592177], [3.4999515623076847, 203.15712578122046, 0.0, 0.0, 0.0, 0.0, 0.0, 0.0, 0.0, 0.0, 245.276002, 3405677999.5117674], [3.5000293711339054, 203.55975147733406, 0.0, 0.0, 0.0, 0.0, 0.0, 0.0, 0.0, 0.0, 246.571982, 3405678016.8942432], [3.499928695230804, 203.95987935488316, 0.0, 0.0, 0.0, 0.0, 0.0, 0.0, 0.0, 0.0, 247.643846, 3405678034.950854], [3.4999810452343882, 204.35421169153307, 0.0, 0.0, 0.0, 0.0, 0.0, 0.0, 0.0, 0.0, 248.79995599999998, 3405678052.6083846], [3.500253306905088, 204.7668519105477, 0.0, 0.0, 0.0, 0.0, 0.0, 0.0, 0.0, 0.0, 250.06435800000003, 3405678070.215905], [3.50009289505293, 205.16224731117572, 0.0, 0.0, 0.0, 0.0, 0.0, 0.0, 0.0, 0.0, 251.000746, 3405678087.837429], [3.500043884753447, 205.55500827630178, 0.0, 0.0, 0.0, 0.0, 0.0, 0.0, 0.0, 0.0, 252.13923, 3405678105.229907], [3.5001887541816945, 205.96445886297474, 0.0, 0.0, 0.0, 0.0, 0.0, 0.0, 0.0, 0.0, 252.97609799999998, 3405678122.979456], [3.4998946087703846, 206.35566420180572, 0.0, 0.0, 0.0, 0.0, 0.0, 0.0, 0.0, 0.0, 253.46864, 3405678140.617983], [3.500150624544607, 206.7587565036897, 0.0, 0.0, 0.0, 0.0, 0.0, 0.0, 0.0, 0.0, 254.25409000000002, 3405678158.314522], [3.500372440769697, 207.17307899982382, 0.0, 0.0, 0.0, 0.0, 0.0, 0.0, 0.0, 0.0, 254.860408, 3405678176.085075], [3.5002043029657575, 207.56618854110292, 0.0, 0.0, 0.0, 0.0, 0.0, 0.0, 0.0, 0.0, 255.312016, 3405678194.047667], [3.500198333823385, 207.96656790708536, 0.0, 0.0, 0.0, 0.0, 0.0, 0.0, 0.0, 0.0, 255.840796, 3405678211.797216], [3.499951551950398, 208.3575457829392, 0.0, 0.0, 0.0, 0.0, 0.0, 0.0, 0.0, 0.0, 256.10305400000004, 3405678229.4327426], [3.500083282951993, 208.76417733595747, 0.0, 0.0, 0.0, 0.0, 0.0, 0.0, 0.0, 0.0, 256.365226, 3405678247.1622877], [3.500124885329094, 209.16025699143526, 0.0, 0.0, 0.0, 0.0, 0.0, 0.0, 0.0, 0.0, 256.449384, 3405678265.2018948], [3.500280507445082, 209.5620715582811, 0.0, 0.0, 0.0, 0.0, 0.0, 0.0, 0.0, 0.0, 256.606032, 3405678283.0854707], [3.5001355349900383, 209.96319017558017, 0.0, 0.0, 0.0, 0.0, 0.0, 0.0, 0.0, 0.0, 256.648488, 3405678300.678989], [3.5000367357214985, 210.3566080720418, 0.0, 0.0, 0.0, 0.0, 0.0, 0.0, 0.0, 0.0, 256.668226, 3405678318.796612], [3.500262261288431, 210.76657422280746, 0.0, 0.0, 0.0, 0.0, 0.0, 0.0, 0.0, 0.0, 256.41913999999997, 3405678336.5571632], [3.50001765614118, 211.16395661768834, 0.0, 0.0, 0.0, 0.0, 0.0, 0.0, 0.0, 0.0, 256.23910800000004, 3405678354.4047318], [3.500095413842314, 211.5607876383894, 0.0, 0.0, 0.0, 0.0, 0.0, 0.0, 0.0, 0.0, 255.877226, 3405678372.1272755], [3.4999688394327175, 211.96080448756484, 0.0, 0.0, 0.0, 0.0, 0.0, 0.0, 0.0, 0.0, 255.823436, 3405678389.6097713], [3.5001210085509906, 212.36087184530203, 0.0, 0.0, 0.0, 0.0, 0.0, 0.0, 0.0, 0.0, 255.592128, 3405678407.450339], [3.500094706847231, 212.76047437984866, 0.0, 0.0, 0.0, 0.0, 0.0, 0.0, 0.0, 0.0, 255.17608199999998, 3405678425.866021], [3.500107533805212, 213.1663546938393, 0.0, 0.0, 0.0, 0.0, 0.0, 0.0, 0.0, 0.0, 18.894842, 3405678443.743596], [3.499981066020215, 213.5626663942656, 0.0, 0.0, 0.0, 0.0, 0.0, 0.0, 0.0, 0.0, 21.59437, 3405678461.8342133], [3.5000185085939197, 213.9562638610255, 0.0, 0.0, 0.0, 0.0, 0.0, 0.0, 0.0, 0.0, 22.61374, 3405678479.2636986], [3.500040125555706, 214.3605841191766, 0.0, 0.0, 0.0, 0.0, 0.0, 0.0, 0.0, 0.0, 23.058656000000003, 3405678497.258297], [3.499802393564528, 214.75924494385148, 0.0, 0.0, 0.0, 0.0, 0.0, 0.0, 0.0, 0.0, 22.982956, 3405678514.8748193], [3.499803939265741, 215.16354345707683, 0.0, 0.0, 0.0, 0.0, 0.0, 0.0, 0.0, 0.0, 23.229728, 3405678532.8584156], [3.500369141804904, 215.56688575866002, 0.0, 0.0, 0.0, 0.0, 0.0, 0.0, 0.0, 0.0, 23.424183999999997, 3405678550.5779586], [3.500161803245673, 215.9657417759897, 0.0, 0.0, 0.0, 0.0, 0.0, 0.0, 0.0, 0.0, 23.930082, 3405678568.319506], [3.500235825440909, 216.37263028223322, 0.0, 0.0, 0.0, 0.0, 0.0, 0.0, 0.0, 0.0, 24.551527999999998, 3405678586.157073], [3.500391494361738, 216.76838082664366, 0.0, 0.0, 0.0, 0.0, 0.0, 0.0, 0.0, 0.0, 25.711326, 3405678604.0446496], [3.5002297132188342, 217.16906156084514, 0.0, 0.0, 0.0, 0.0, 0.0, 0.0, 0.0, 0.0, 27.227771999999998, 3405678621.9252253], [3.4999849230532414, 217.5587106962735, 0.0, 0.0, 0.0, 0.0, 0.0, 0.0, 0.0, 0.0, 29.497405999999998, 3405678640.1158624], [3.4999994805285333, 217.96002396771559, 0.0, 0.0, 0.0, 0.0, 0.0, 0.0, 0.0, 0.0, 31.977788, 3405678657.8634114], [3.499803830002476, 218.36396625714346, 0.0, 0.0, 0.0, 0.0, 0.0, 0.0, 0.0, 0.0, 33.175976, 3405678675.825003], [3.499967860566722, 218.76675184546426, 0.0, 0.0, 0.0, 0.0, 0.0, 0.0, 0.0, 0.0, 33.601279999999996, 3405678693.7665906], [3.499996189626497, 219.16768390175494, 0.0, 0.0, 0.0, 0.0, 0.0, 0.0, 0.0, 0.0, 34.236796, 3405678711.6301627], [3.500094284515776, 219.5604087360409, 0.0, 0.0, 0.0, 0.0, 0.0, 0.0, 0.0, 0.0, 34.145070000000004, 3405678729.4327226], [3.500180948936783, 219.96596929542105, 0.0, 0.0, 0.0, 0.0, 0.0, 0.0, 0.0, 0.0, 33.620538, 3405678747.0712495], [3.4998848304622827, 220.36099409149014, 0.0, 0.0, 0.0, 0.0, 0.0, 0.0, 0.0, 0.0, 33.671206, 3405678764.7207785], [3.5001638170805665, 220.76758978679683, 0.0, 0.0, 0.0, 0.0, 0.0, 0.0, 0.0, 0.0, 33.419056000000005, 3405678782.4793296], [3.5001243371200403, 221.16683007914466, 0.0, 0.0, 0.0, 0.0, 0.0, 0.0, 0.0, 0.0, 32.855821999999996, 3405678800.563946], [3.5001110920940786, 221.5666145897472, 0.0, 0.0, 0.0, 0.0, 0.0, 0.0, 0.0, 0.0, 31.902988, 3405678818.4105144], [3.5002429519391933, 221.9676357181876, 0.0, 0.0, 0.0, 0.0, 0.0, 0.0, 0.0, 0.0, 30.553368000000003, 3405678836.3691053], [3.4998570388088712, 222.36449608450104, 0.0, 0.0, 0.0, 0.0, 0.0, 0.0, 0.0, 0.0, 28.834168, 3405678853.7825875], [3.4997816518320115, 222.76394903933627, 0.0, 0.0, 0.0, 0.0, 0.0, 0.0, 0.0, 0.0, 26.935568000000004, 3405678871.716173]]
  in  "Notes:":string="Datum: 2.12.11, Uhrzeit: 13:03, T0.3K,PID LOOPP 0.2, I  200: , Filter auf 12dB und 30Hz, PID Dämpfung:  P=0.5, D=6.2E-5, Laser 25°, 20mA, AOM 10mA, Sweep 0.15T/min,Winkelsweep 0.4° Winkelschritte, warten bei jedem Feldpunkt (measurevsB2Dv8.vi))4s, vectorsm1.txt,Kryo auf dem Boden,mit neuem PS, großer Abstand zwischen Faser und Cantilever(3V Signalamplitude), automatisches Umschalten des Feedbackdämpfung" caption="Notizen:"
  out "Messfile Refnum":refnum<file>
  in  "Measurement File":path=path "D:/UserData/Matthias/Messungen/STO_LAOR103/111202/111202_R103_anglesweep_3,5T_1.txt"
  in  "Sample name:":string="R103"
  in  "HP 1":bool=TRUE
  in  "GPIB HP":string="14"
  in  "HP 2":bool
  in  "LI 3":bool
  in  "GPIB L 3":string="8"
  in  "LI 2":bool
  in  "GPIB L 2":string="8"
  in  "LI 1":bool
  in  "GPIB L 1":string="8"
  out "Number of lines":i32=2320
  in  "Operation":u16(ring)=1 items=["Stepwise", "Continous"]
  out "Ramp Rate along Vector (T/min)":dbl=0.15 format="%.3f"
  out "Current Ramp Rate Z (T/min)":dbl=0.10976056469738536 format="%.3f"
  out "Current Ramp Rate Y (T/min)":dbl=0.10223804789466143 format="%.3f"
  in  "User defined Ramp Rate (T/min)":bool=TRUE
  in  "User defined Ramp Rate (T/min)":dbl=0.15 format="%.3f"
  in  "Z-Axis Communications Config":T3={"GPIB address"=22, "GPIB bus"=1, "connection ID"=refnum, "IP"="111.111.111.1", "Active Comm Interface"=0, "Serial Port"="", "Programmer Type"=0} {"Programmer Type" items=["Model 430", "Model 420"]; "Active Comm Interface" items=["TCP/IP (Model 430 Only)", "RS232", "IEEE488"]}
  in  "Max Ramp Rate - Y Axis (A/s)":dbl=0.055 format="%.3f"
  in  "Max Ramp Rate - Z Axis (A/s)":dbl=0.19 format="%.3f"
  in  "Magnitude Limit (kG)":dbl=45.1 format="%.3f"
  in  "Y-Axis Communications Config":T3={"GPIB address"=22, "GPIB bus"=1, "connection ID"=refnum, "IP"="111.111.111.2", "Active Comm Interface"=0, "Serial Port"="", "Programmer Type"=0} {"Programmer Type" items=["Model 430", "Model 420"]; "Active Comm Interface" items=["TCP/IP (Model 430 Only)", "RS232", "IEEE488"]}
  out "Cartesian Display (T)":T4={"Y-Axis Field (T)"=0.01746, "Z-Axis Field (T)"=0.99986} {"Z-Axis Field (T)" format="%.3f"; "Y-Axis Field (T)" format="%.3f"}
  in  "Starting index":i32=334
  in  "Normal color":u32(colorbox)=11711154
  in  "Highlight color":u32(colorbox)=16711680
  in  "Prompt for File?":bool
  out "Continue Execution?":bool=TRUE
  out "error out":T5
  in  "error in":T5
  out "STATUS":string="Zeroing vector."
  in  "Ramping Control":u16(ring)=4 items=["NEXT VECTOR", "RAMPING", "HOLDING", "PAUSE", "ZERO"]
  out "Cartesian Display (kG)":T6 {"Z-Axis Field (kG)" format="%.3f"; "Y-Axis Field (kG)" format="%.3f"}
  in  "Field Values":string[][](table)=array2320x2[4640 elements]
  out "Switch Heaters":bool=TRUE
  out "Polar Display (T)":T7 {"Field Magnitude (T)" format="%.3f"; "q (degrees)" format="%.3f"}
  out "Polar Display (kG)":T8 {"Field Magnitude (kG)" format="%.3f"; "q (degrees)" format="%.3f"}
  in  "Coordinate System":u16(ring)=1 items=["Cartesian", "Polar"]
  in  "Magnetic Field Units":u16(ring)=1 items=["kG", "Tesla"]
  # "Measurement Display"
  # "Measurement Settings"
  # "Magnet Settings"
  # "Max Ramp Rate z: 1.27 T/min\nMax Ramp Rate y: 0.17 T/min"
  # "Devices"
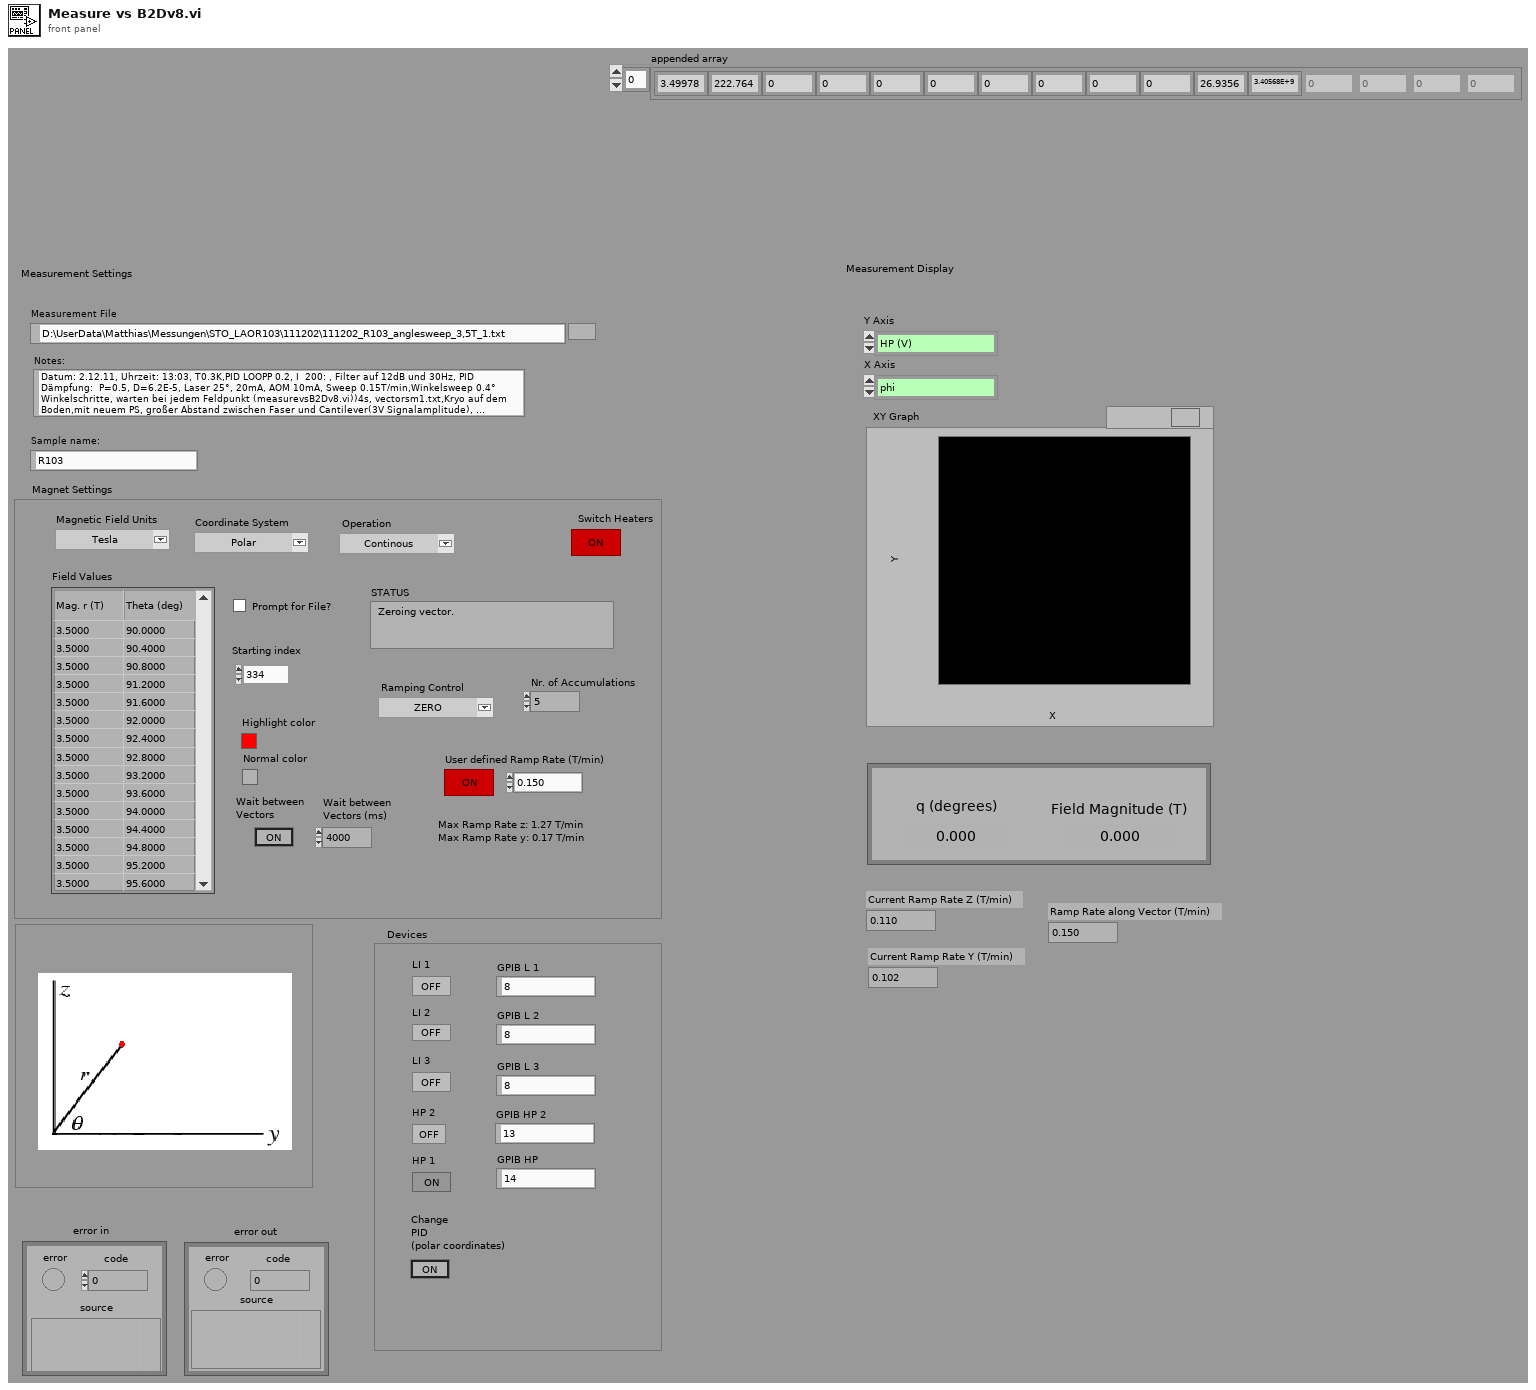
[diagram p1: front panel]
types:
  T1 = enum16{"B", "phi", "LI 1 Vx", "LI 1 phase", "LI 2 Vx", "LI 2 phase", "LI 3 Vx", "LI 3 phase", "LI 4 Vx", "LI 4 phase", "HP (V)"}
  T2 = cluster{"measured data":dbl[], "measured data":dbl[]}
  T3 = cluster{"GPIB address":i16, "GPIB bus":i16, "connection ID":refnum<k5>, "IP":string, "Active Comm Interface":u16, "Serial Port":refnum<visa-resource-name>, "Programmer Type":u16}
  T4 = cluster{"Y-Axis Field (T)":dbl, "Z-Axis Field (T)":dbl}
  T5 = cluster{"error":bool, "code":i32, "source":string}
  T6 = cluster{"Y-Axis Field (kG)":dbl, "Z-Axis Field (kG)":dbl}
  T7 = cluster{"q (degrees)":dbl, "Field Magnitude (T)":dbl}
  T8 = cluster{"q (degrees)":dbl, "Field Magnitude (kG)":dbl}
  T9 = enum16{"", "RAMPING", "HOLDING", "PAUSED", "MANUAL UP", "MANUAL DOWN", "ZEROING CURRENT", "QUENCH DETECTED", "HEATING SWITCH"}
  T10 = enum16{"", "RAMPING", "HOLDING", "PAUSED", "MANUAL UP", "MANUAL DOWN", "ZEROING CURRENT", "QUENCH DETECTED", "HEATING SWITCH", "AT ZER0", "COOLING SWITCH"}
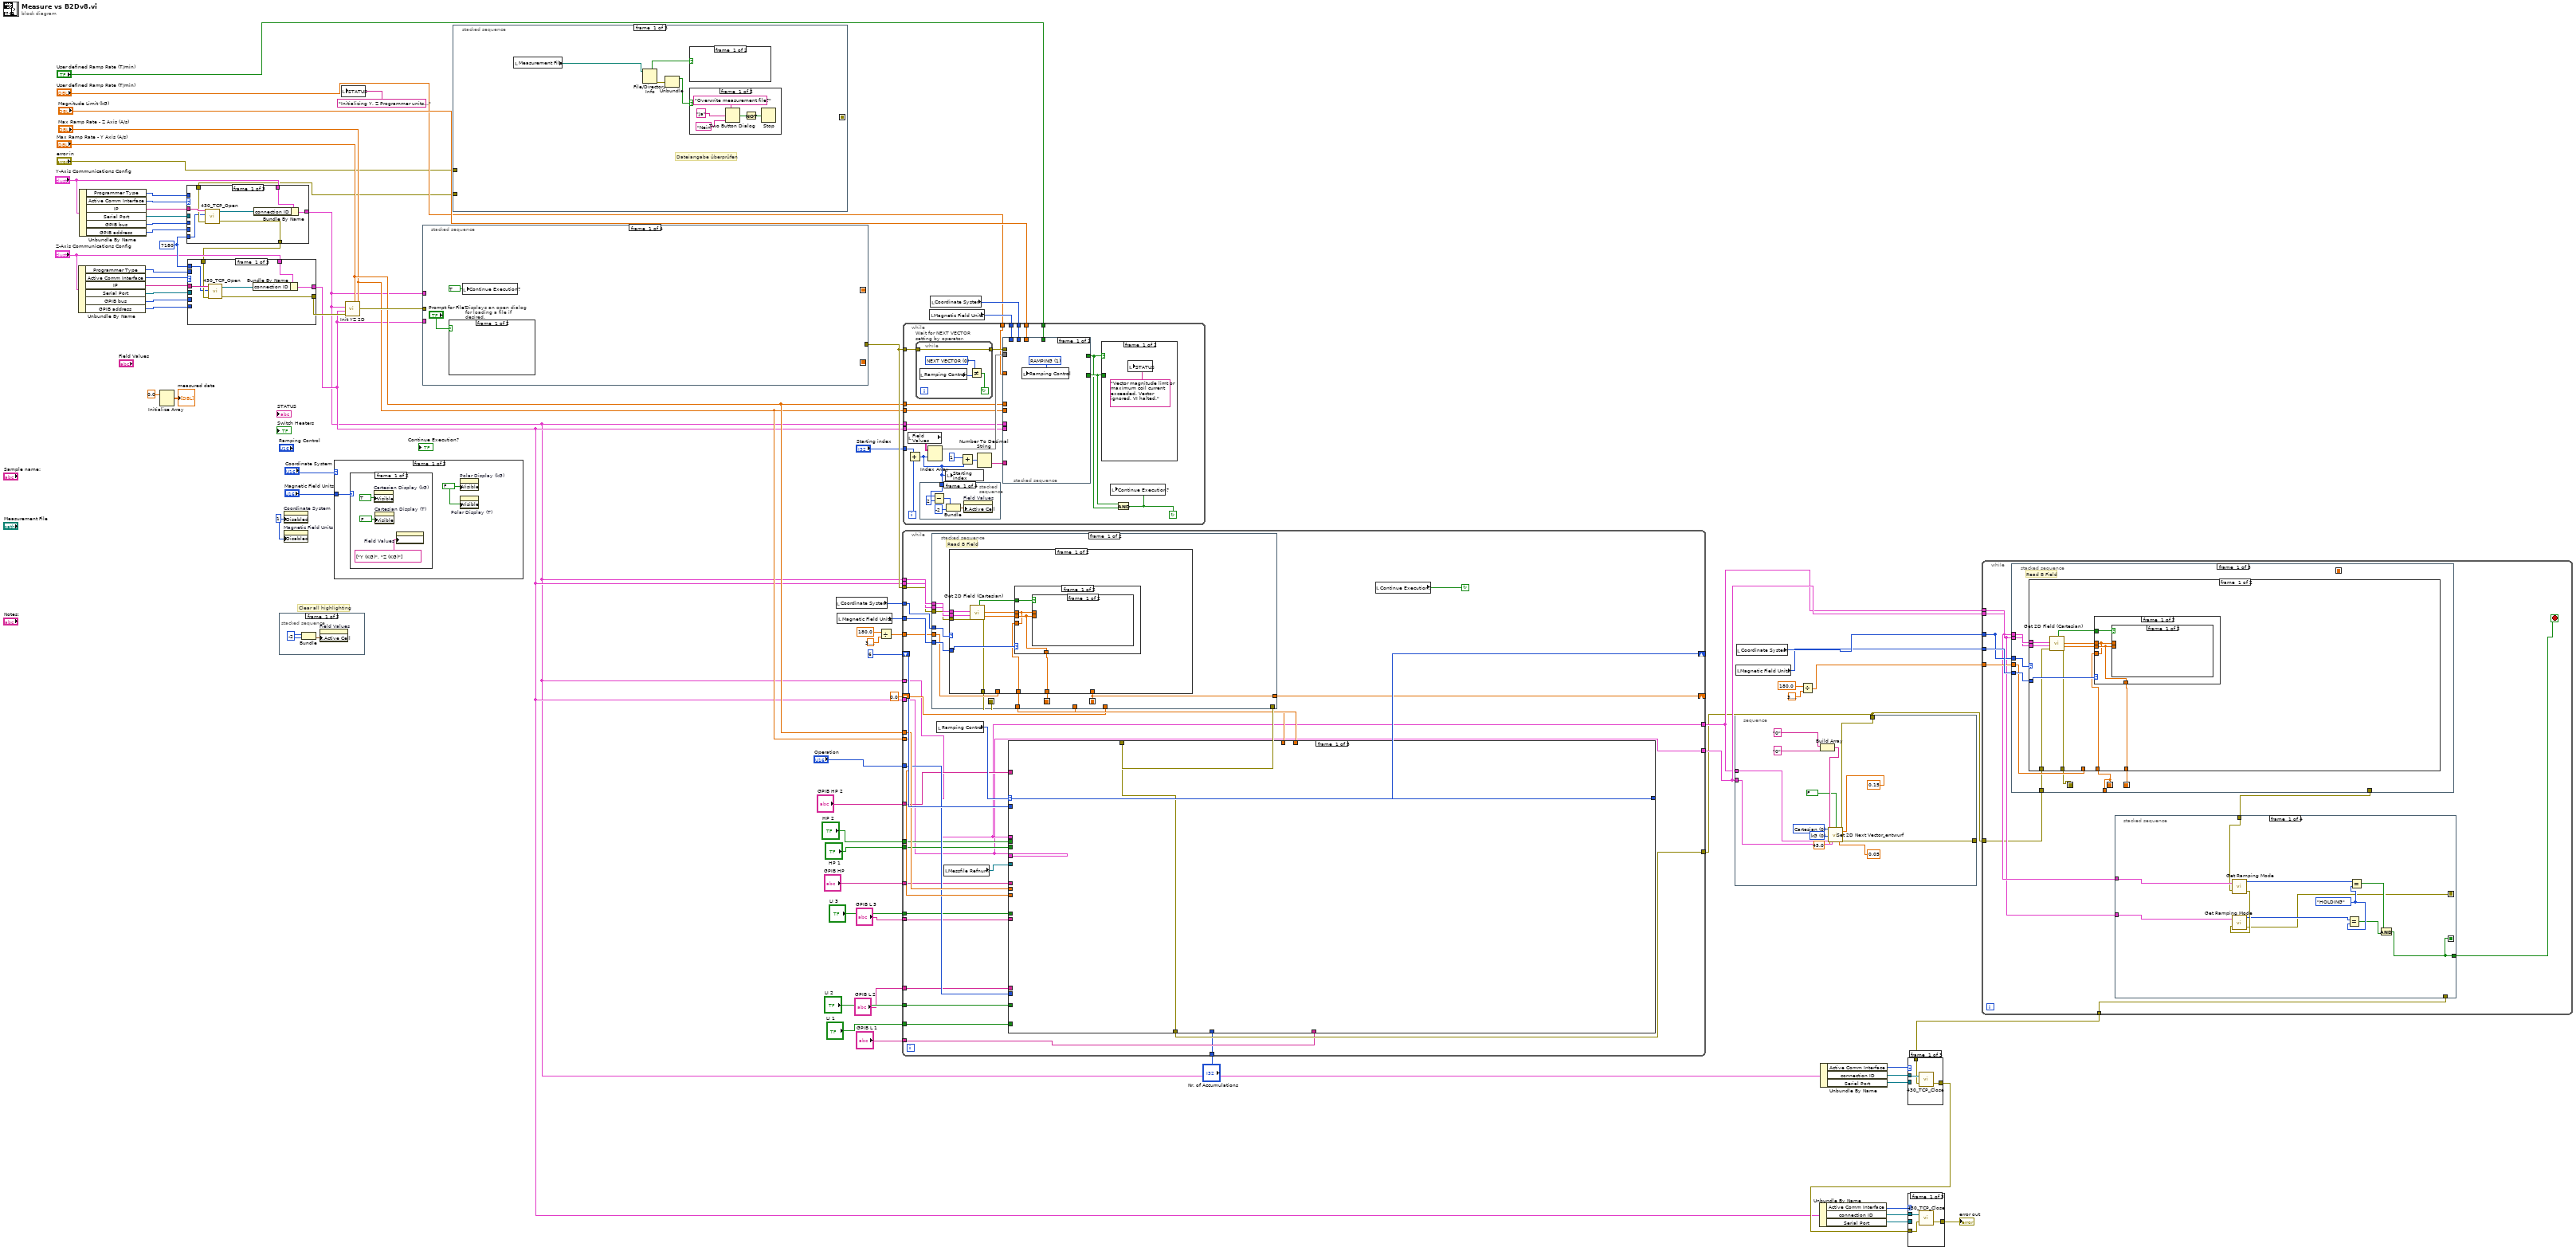
[diagram p0: block diagram]
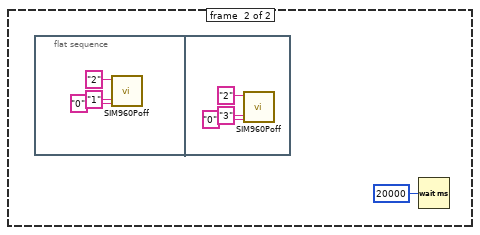
[diagram p3: hidden frame]
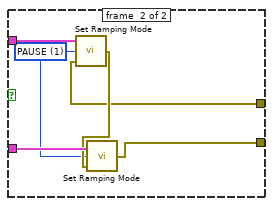
[diagram p5: hidden frame]
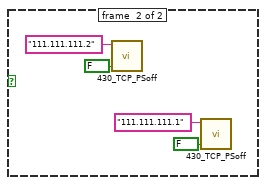
[diagram p7: hidden frame]
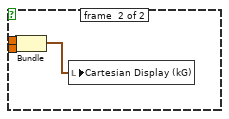
[diagram p8: hidden frame]
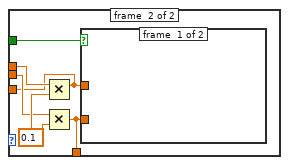
[diagram p9: hidden frame]
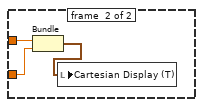
[diagram p10: hidden frame]
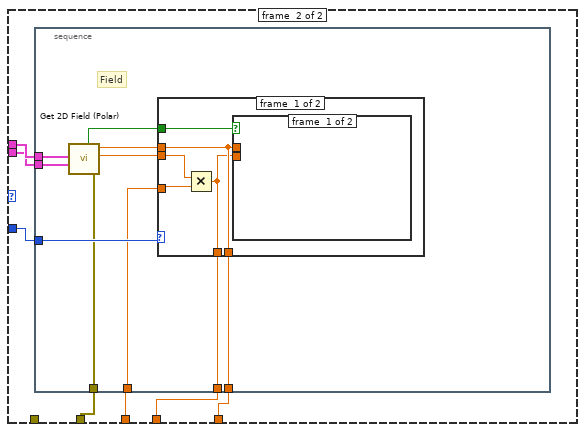
[diagram p11: hidden frame]
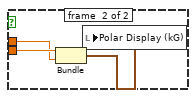
[diagram p12: hidden frame]
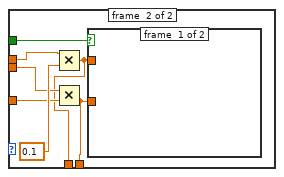
[diagram p13: hidden frame]
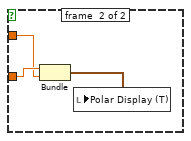
[diagram p14: hidden frame]
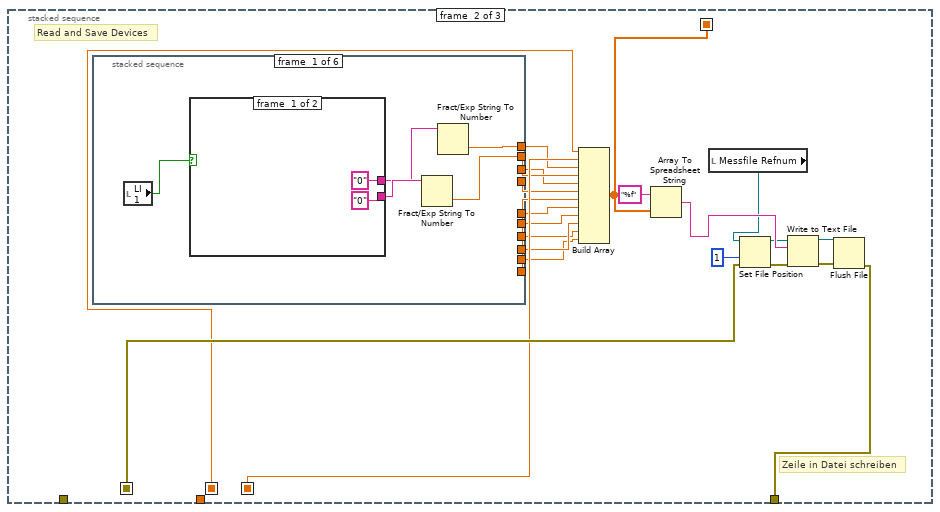
[diagram p15: hidden frame]
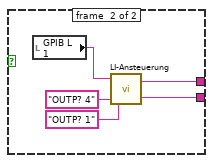
[diagram p16: hidden frame]
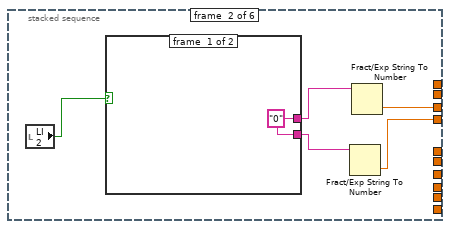
[diagram p17: hidden frame]
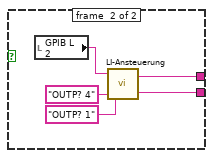
[diagram p18: hidden frame]
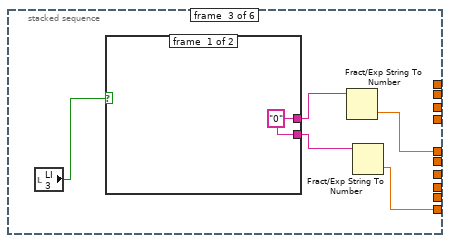
[diagram p19: hidden frame]
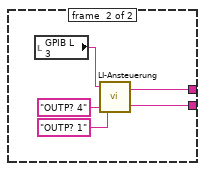
[diagram p20: hidden frame]
diagram:
  w58 = 7180 ("TCP Port")
  w71 = u8 1 ("Write Attribute")
  # "Clear all highlighting"
  n1 = Unbundle By Name("Z-Axis Communications Config") -> ("Programmer Type"=w37:u16, "Active Comm Interface"=w57:u16, "IP"=w54:string, "Serial Port"=w53:refnum<visa-resource-name>, "GPIB bus"=w36:i16, "GPIB address"=w35:i16)
  n2 = Unbundle By Name("Y-Axis Communications Config") -> ("Programmer Type"=w31:u16, "Active Comm Interface"=w56:u16, "IP"=w55:string, "Serial Port"=w52:refnum<visa-resource-name>, "GPIB bus"=w32:i16, "GPIB address"=w33:i16)
  n3 = Initialize Array(0.0 ("element")) -> (→"measured data":dbl[][])  [unwired: 2 in]
  n4 = stacked-sequence {
    frame #0 {
      w74 = -2
      n5 = Bundle(w74, w74) -> (w75:cluster{i32, i32})  [unwired: 1 in]
      n6 = property on="Field Values" class="Tbl (strict)"("Active Cell:Active Cell"=w75) -> ()  [unwired: 2 in, 2 out]
    }
    frame #1 {
      n7 = property on="Field Values" class="Tbl (strict)"("Active Cell:Cell Background Color"="Normal color") -> ()  [unwired: 2 in, 2 out]
    }
  }
  n8 = property on="Coordinate System" class="Ring (strict)"("Disabled"=w71) -> ()  [unwired: 2 in, 2 out]
  n9 = property on="Magnetic Field Units" class="Ring (strict)"("Disabled"=w71) -> ()  [unwired: 2 in, 2 out]
  n10 = case shown="0, Default" "Coordinate System" {
    tunnel: "Magnetic Field Units" -> [w78 w86]
    frame #0 {
      w77 = FALSE ("Write Attribute")
      (unwired) FALSE ("Write Attribute")
      (unwired) TRUE ("Write Attribute")
      n11 = case shown="1" w78 {
        frame #0 {
          n12 = property on="Cartesian Display (kG)" class="Cluster (strict)"("Visible"=TRUE ("Write Attribute")) -> ()  [unwired: 2 in, 2 out]
          n13 = property on="Cartesian Display (T)" class="Cluster (strict)"("Visible"=FALSE ("Write Attribute")) -> ()  [unwired: 2 in, 2 out]
          n14 = property on="Field Values" class="Tbl (strict)"("Column Header Strings[]"=string[] ["Y (KG)", "Z (KG)"] ("Write Attribute")) -> ()  [unwired: 2 in, 2 out]
        }
        frame #1 {
          n15 = property on="Cartesian Display (kG)" class="Cluster (strict)"("Visible"=FALSE ("Write Attribute")) -> ()  [unwired: 2 in, 2 out]
          n16 = property on="Cartesian Display (T)" class="Cluster (strict)"("Visible"=TRUE ("Write Attribute")) -> ()  [unwired: 2 in, 2 out]
          n17 = property on="Field Values" class="Tbl (strict)"("Column Header Strings[]"=string[] ["Y (T)", "Z (T)"] ("Write Attribute")) -> ()  [unwired: 2 in, 2 out]
        }
      }
      n18 = property on="Polar Display (kG)" class="Clust (strict)"("Visible"=w77) -> ()  [unwired: 2 in, 2 out]
      n19 = property on="Polar Display (T)" class="Clust (strict)"("Visible"=w77) -> ()  [unwired: 2 in, 2 out]
    }
    frame #1 {
      (unwired) FALSE ("Write Attribute")
      (unwired) TRUE ("Write Attribute")
      w85 = FALSE ("Write Attribute")
      n20 = case shown="1" w86 {
        frame #0 {
          n21 = property on="Polar Display (kG)" class="Clust (strict)"("Visible"=TRUE ("Write Attribute")) -> ()  [unwired: 2 in, 2 out]
          n22 = property on="Polar Display (T)" class="Clust (strict)"("Visible"=FALSE ("Write Attribute")) -> ()  [unwired: 2 in, 2 out]
          n23 = property on="Field Values" class="Tbl (strict)"("Column Header Strings[]"=string[] ["Mag. r (KG)", "Theta (deg)"] ("Write Attribute")) -> ()  [unwired: 2 in, 2 out]
        }
        frame #1 {
          n24 = property on="Polar Display (kG)" class="Clust (strict)"("Visible"=FALSE ("Write Attribute")) -> ()  [unwired: 2 in, 2 out]
          n25 = property on="Polar Display (T)" class="Clust (strict)"("Visible"=TRUE ("Write Attribute")) -> ()  [unwired: 2 in, 2 out]
          n26 = property on="Field Values" class="Tbl (strict)"("Column Header Strings[]"=string[] ["Mag. r (T)", "Theta (deg)"] ("Write Attribute")) -> ()  [unwired: 2 in, 2 out]
        }
      }
      n27 = property on="Cartesian Display (kG)" class="Cluster (strict)"("Visible"=w85) -> ()  [unwired: 2 in, 2 out]
      n28 = property on="Cartesian Display (T)" class="Cluster (strict)"("Visible"=w85) -> ()  [unwired: 2 in, 2 out]
    }
  }
  n29 = local write "STATUS"("Initializing Y, Z Programmer units..." ("STATUS")) -> ()
  n30 = stacked-sequence {
    seq-local: [_ w104 _] -> [_ _ w123]
    tunnel: "error in" -> [_ w105 _]
    tunnel: [_ _ w122] -> w26
    frame #0 {
      # "Dateiangabe überprüfen"
      n31 = local read "Measurement File"() -> (w96:path)
      n32 = File/Directory Info(path=w96) -> (directory=w94:bool, error out=w95:errorcluster)  [unwired: 1 in, 5 out]
      n33 = Unbundle(w95) -> ("status"=w93:bool)  [unwired: 2 out]
      n34 = case shown="False" w94 {
        frame #0 {
        }
        frame #1 {
          n35 = One Button Dialog(message="Invalid\nfilename!") -> (true=w102:bool)  [unwired: 1 in]
          n36 = Stop(stop? (T)=w102) -> ()
        }
      }
      n37 = case shown="False" w93 {
        frame #0 {
          n38 = Two Button Dialog(message="Overwrite measurement file?", 1:"Nein", 2:"Ja") -> (T button?=w98:bool)
          n39 = Not(x=w98) -> (.not. x?=w97:bool)
          n40 = Stop(stop? (T)=w97) -> ()
        }
        frame #1 {
        }
      }
    }
    frame #1 {
      w108 = "\r"
      # "Erstellen\ndes Headers"
      n41 = local read "User defined Ramp Rate (T/min)"() -> (w107:dbl)
      n42 = local read "Sample name:"() -> (w114:string)
      n43 = local read "Notes:"() -> (w116:string)
      n44 = Get Date/Time In Seconds() -> (seconds since 1Jan1904=w110:timestamp)
      n45 = Get Date/Time String(seconds (now)=w110) -> (date string=w112:string)  [unwired: 2 in, 1 out]
      n46 = Number To Fractional String(number=w107) -> (F-format string=w106:string)  [unwired: 3 in]
      n47 = Concatenate Strings("Date: ", w112, w108, "Sample name: ", w114, w108, "Notes: ", w116, w108, "Sweeprate: ", w106, w108) -> (w120:string)
      n48 = local read "Measurement File"() -> (w117:path)
      n49 = Open/Create/Replace File(file path (use dialog)=w117, error in=w105, operation (0:open)=4) -> (refnum out=w119:refnum<file>, error out=w121:errorcluster)  [unwired: 3 in, 1 out]
      "Messfile Refnum" <- w119
      n50 = Write to Text File(file (use dialog)=w119, text=w120, error in=w121) -> (error out=w104:errorcluster)  [unwired: 1 in, 2 out]
    }
    frame #2 {
      w126 = "\t"
      w124 = "\r"
      # "Erstellen der Spalten-\nbeschriftungen"
      n51 = local read "Messfile Refnum"() -> (w133:refnum<file>)
      n52 = Set File Position(refnum=w133, from (0:start)=1, error in=w123) -> (refnum out=w139:refnum<file>, error out=w141:errorcluster)  [unwired: 1 in]
      n53 = Concatenate Strings(w124, "B-Field Y/R", w126, "B-Field Z/phi", w126, "LI 1 Vx", w126, "LI 1 Vy", w126, "LI 2 Vx", w126, "LI 2 Vy", w126, "LI 3 Vx", w126, "LI 3 Vy", w126, "LI 4 Vx", w126, "LI 4 Vy", w126, "HP (V)", w126, "Timestamp", w124) -> (w140:string)
      n54 = Write to Text File(file (use dialog)=w139, text=w140, error in=w141) -> (refnum out=w143:refnum<file>, error out=w142:errorcluster)  [unwired: 1 in, 1 out]
      n55 = Flush File(refnum=w143, error in=w142) -> (error out=w122:errorcluster)  [unwired: 1 out]
    }
  }
  n56 = case shown="2" w56 {
    tunnel: w55 -> [w151 _ _]
    tunnel: w26 -> [w150 w157 w159]
    tunnel: "Y-Axis Communications Config" -> [w149 w152 w163]
    tunnel: [w147 w155 w163] -> w10
    tunnel: [w146 w156 w158] -> w34
    tunnel: w58 -> [w145 _ _]
    tunnel: w52 -> [_ w153 _]
    tunnel: w33 -> [_ _ w162]
    tunnel: w32 -> [_ _ w161]
    tunnel: w31 -> [_ _ w160]
    frame #0 {
      n57 = call <userlib>:"430_TCP_Open.vi"("IP Address"=w151, "TCP Port"=w145, "error in (no error)"=w150) -> ("connection ID"=w148:refnum<k5>, "error out"=w146:errorcluster)  [unwired: 3 in, 1 out]
      n58 = Bundle By Name(cluster=w149, "connection ID"=w148) -> (w147:T3)
    }
    frame #1 {
      n59 = call <userlib>:"430_RS232_Open.vi"("VISA resource name"=w153, "error in (no error)"=w157) -> ("VISA resource name out"=w154:refnum<visa-resource-name>, "error out"=w156:errorcluster)  [unwired: 5 in]
      n60 = Bundle By Name(cluster=w152, "Serial Port"=w154) -> (w155:T3)
    }
    frame #2 {
      n61 = case shown="0, Default" w160 {
        tunnel: w161 -> [w167 _]
        tunnel: w162 -> [w166 _]
        tunnel: w159 -> [w165 w168]
        tunnel: [w164 w168] -> w158
        frame #0 {
          n62 = DevClear(2:w165, 3:w166, 4:w167) -> (0:w164:errorcluster)  [unwired: 1 out]
        }
        frame #1 {
        }
      }
    }
  }
  n63 = case shown="2" w57 {
    tunnel: w54 -> [w175 _ _]
    tunnel: w34 -> [w174 w181 w183]
    tunnel: [w173 w180 w182] -> w51
    tunnel: "Z-Axis Communications Config" -> [w172 w178 w187]
    tunnel: [w170 w179 w187] -> w11
    tunnel: w58 -> [w169 _ _]
    tunnel: w53 -> [_ w176 _]
    tunnel: w37 -> [_ _ w186]
    tunnel: w36 -> [_ _ w185]
    tunnel: w35 -> [_ _ w184]
    frame #0 {
      n64 = call <userlib>:"430_TCP_Open.vi"("IP Address"=w175, "TCP Port"=w169, "error in (no error)"=w174) -> ("connection ID"=w171:refnum<k5>, "error out"=w173:errorcluster)  [unwired: 3 in, 1 out]
      n65 = Bundle By Name(cluster=w172, "connection ID"=w171) -> (w170:T3)
    }
    frame #1 {
      n66 = call <userlib>:"430_RS232_Open.vi"("VISA resource name"=w176, "error in (no error)"=w181) -> ("VISA resource name out"=w177:refnum<visa-resource-name>, "error out"=w180:errorcluster)  [unwired: 5 in]
      n67 = Bundle By Name(cluster=w178, "Serial Port"=w177) -> (w179:T3)
    }
    frame #2 {
      n68 = case shown="0, Default" w186 {
        tunnel: w185 -> [w191 _]
        tunnel: w184 -> [w190 _]
        tunnel: w183 -> [w189 w192]
        tunnel: [w188 w192] -> w182
        frame #0 {
          n69 = DevClear(2:w189, 3:w190, 4:w191) -> (0:w188:errorcluster)  [unwired: 1 out]
        }
        frame #1 {
        }
      }
    }
  }
  n70 = call <userlib>:"Init YZ 2D.vi"("Max Ramp Rate Z-axis"="Max Ramp Rate - Z Axis (A/s)", "Max Ramp Rate Y-axis"="Max Ramp Rate - Y Axis (A/s)", "error in"=w51, "Z-Axis Communications Config"=w11, "Y-Axis Communications Config"=w10) -> ("error out"=w69:T5)  [unwired: 5 in]
  n71 = stacked-sequence {
    seq-local: [_ w200 _ _] -> [_ _ w247 _]
    seq-local: [_ w199 _ _] -> [_ _ w246 _]
    tunnel: w11 -> [_ w202 _ _]
    tunnel: w69 -> [_ w203 _ _]
    tunnel: [_ w198 _ _] -> w65
    tunnel: w10 -> [_ w201 _ _]
    frame #0 {
      n72 = case "Displays an open dialog for loading a file if desired." shown="True" "Prompt for File?" {
        frame #0 {
        }
        frame #1 {
          n73 = call-poly <vilib>:"Read From Spreadsheet File.vi"() -> ("all rows"=w197:dbl[][])  [unwired: 7 in, 4 out]
          n74 = Number To Fractional String(number=w197, precision (6)=i16 4) -> (F-format string=w196:string[][])  [unwired: 2 in]
          n75 = local write "Field Values"(w196) -> ()
        }
      }
      n76 = local write "Continue Execution?"(TRUE ("Continue Execution?")) -> ()
    }
    frame #1 {
      w211 = u16 3 items=["NEXT VECTOR", "RAMPING", "HOLDING", "PAUSE", "ZERO"] ("Ramping Control")
      n77 = call <userlib>:"Get Switch Present.vi"("error in"=w203, "Communications Config"=w201) -> ("error out"=w207:T5, "Switch Present?"=w208:bool)
      n78 = case shown="True" w208 {
        tunnel: w207 -> [w229 w238]
        tunnel: w201 -> [_ w231]
        tunnel: [0.0 w235] -> w199
        tunnel: [w229 w237] -> w206
        frame #0 {
        }
        frame #1 {
          n79 = call <userlib>:"Get Switch Heater Time.vi"("error in"=w238, "Communications Config"=w231) -> ("error out"=w234:T5, "Switch Heating Time (secs)"=w236:dbl)
          n80 = call <userlib>:"Get Switch Heater.vi"("error in"=w234, "Communications Config"=w231) -> ("error out"=w233:T5, "Switch Heater Indicator"=w232:bool)
          n81 = case shown="False" w232 {
            tunnel: [w243 w244] -> w237
            tunnel: w236 -> [w241 _]
            tunnel: [w241 0.0] -> w235
            tunnel: w233 -> [w239 w244]
            tunnel: w231 -> [w240 _]
            frame #0 {
              n82 = call <userlib>:"Set Switch Heater.vi"("error in"=w239, "Switch Heater Control"=TRUE, "Communications Config"=w240) -> ("error out"=w243:T5)
            }
            frame #1 {
            }
          }
        }
      }
      n83 = call <userlib>:"Get Switch Present.vi"("error in"=w206, "Communications Config"=w202) -> ("error out"=w204:T5, "Switch Present?"=w205:bool)
      n84 = case shown="True" w205 {
        tunnel: w204 -> [w212 w221]
        tunnel: w202 -> [_ w214]
        tunnel: [0.0 w218] -> w200
        tunnel: [w212 w220] -> w198
        frame #0 {
        }
        frame #1 {
          n85 = call <userlib>:"Get Switch Heater Time.vi"("error in"=w221, "Communications Config"=w214) -> ("error out"=w217:T5, "Switch Heating Time (secs)"=w219:dbl)
          n86 = call <userlib>:"Get Switch Heater.vi"("error in"=w217, "Communications Config"=w214) -> ("error out"=w216:T5, "Switch Heater Indicator"=w215:bool)
          n87 = case shown="False" w215 {
            tunnel: [w222 w227] -> w220
            tunnel: w219 -> [w225 _]
            tunnel: [w225 0.0] -> w218
            tunnel: w216 -> [w223 w227]
            tunnel: w214 -> [w224 _]
            frame #0 {
              n88 = call <userlib>:"Set Switch Heater.vi"("error in"=w223, "Switch Heater Control"=TRUE, "Communications Config"=w224) -> ("error out"=w222:T5)
            }
            frame #1 {
            }
          }
        }
      }
      n89 = local write "Ramping Control"(w211) -> ()
      n90 = local write "Switch Heaters"(TRUE ("Switch Heater Control")) -> ()
      n91 = property on="Switch Heaters" class="Boolean (strict)"("Disabled"=u8 1 ("Write Attribute")) -> ()  [unwired: 2 in, 2 out]
    }
    frame #2 {
      n92 = Max & Min(x=w247, y=w246) -> (max(x,y)=w248:dbl)  [unwired: 1 out]
      n93 = local write "STATUS"("Heating switches..." ("STATUS")) -> ()
      n94 = Add(x=w248, y=2) -> (x+y=w252:dbl)
      n95 = property on="Ramping Control" class="Ring (strict)"("Disabled"=u8 1 ("Write Attribute")) -> ()  [unwired: 2 in, 2 out]
      n96 = Multiply(x=w252, y=1000) -> (x*y=w251:dbl)
      n97 = Wait (ms)(milliseconds to wait=w251) -> ()  [unwired: 1 out]
    }
    frame #3 {
      n98 = property on="Ramping Control" class="Ring (strict)"("Disabled"=u8 0 ("Write Attribute")) -> ()  [unwired: 2 in, 2 out]
      n99 = local write "STATUS"("Ready to ramp to first vector. Set Ramping Mode to NEXT VECTOR to begin." ("STATUS")) -> ()
      n100 = local read "Field Values"() -> (w257:string[][])
      n101 = Array Size(array=w257) -> (size(s)=w256:i32[])
      n102 = Index Array(array=w256, index=0) -> (element=→"Number of lines":i32)
    }
  }
  n103 = local read "Coordinate System"() -> (w66:u16)
  n104 = local read "Magnetic Field Units"() -> (w64:u16)
  n105 = Divide(x=180.0, y=3.141592653589793) -> (x/y=w61:dbl)
  n106 = while {
    shift-left: u16 6 ("Ramping Control") -> [w284]
    shift-right: [w285] -> _
    tunnel: [w287] -> w1
    tunnel: w11 -> [w261]
    tunnel: w10 -> [w262]
    tunnel: w61 -> [w289]
    tunnel: w64 -> [w290]
    tunnel: w65 -> [w291]
    tunnel: w11 -> [w292]
    tunnel: w10 -> [w293]
    tunnel: w66 -> [w279]
    tunnel: "Max Ramp Rate - Y Axis (A/s)" -> [w283]
    tunnel: "Max Ramp Rate - Z Axis (A/s)" -> [w282]
    tunnel: "Operation" -> [w281]
    tunnel: "LI 1" -> [w276]
    tunnel: "LI 2" -> [w275]
    tunnel: "LI 3" -> [w274]
    tunnel: "HP 1" -> [w273]
    tunnel: "HP 2" -> [w272]
    tunnel: "GPIB HP" -> [w271]
    tunnel: "GPIB HP 2" -> [w270]
    tunnel: "GPIB L 1" -> [w269]
    tunnel: "GPIB L 2" -> [w268]
    tunnel: "GPIB L 3" -> [w267]
    tunnel: "Nr. of Accumulations" -> [w266]
    shift-right: [w264] -> _
    shift-left: 0.0 -> [w263]
    tunnel: [w262] -> w2
    tunnel: [w261] -> w3
    stop <- w286 continue-if-true
    n107 = stacked-sequence {
      seq-local: [w297 _] -> [_ w369]
      seq-local: [w296 _] -> [_ w370]
      seq-local: [w294 _] -> [_ w368]
      tunnel: w279 -> [w303 _]
      tunnel: w293 -> [w302 _]
      tunnel: w292 -> [w301 _]
      tunnel: w291 -> [w300 _]
      tunnel: w290 -> [w299 _]
      tunnel: w289 -> [w298 _]
      tunnel: [_ w369] -> w280
      tunnel: [_ w370] -> w277
      tunnel: [w295 _] -> w278
      tunnel: [w294 _] -> w264
      tunnel: w263 -> [_ w367]
      frame #0 {
        # "Read B Field"
        n108 = case shown="1" w303 {
          tunnel: w302 -> [w313 w337]
          tunnel: w301 -> [w312 w336]
          tunnel: w300 -> [w311 w335]
          tunnel: w299 -> [w310 w334]
          tunnel: w298 -> [_ w333]
          tunnel: [w306 w332] -> w297
          tunnel: [w305 w330] -> w296
          tunnel: [w304 w331] -> w295
          tunnel: [_ w329] -> w294
          frame #0 {
            n109 = call <userlib>:"Get 2D Field (Cartesian).vi"("Y-Axis Communications Config"=w313, "Z-Axis Communications Config"=w312, "error in"=w311) -> ("All Instruments Responded?"=w307:bool, "Y-Axis Field (kG)"=w309:dbl, "Z-Axis Field (kG)"=w308:dbl, "error out"=w306:T5)  [unwired: 2 in]
            n110 = case shown="1" w310 {
              tunnel: w309 -> [w314 w322]
              tunnel: w308 -> [w315 w323]
              tunnel: w307 -> [w316 w325]
              tunnel: [w315 w321] -> w305
              tunnel: [w314 w320] -> w304
              frame #0 {
                n111 = case shown="True" w316 {
                  tunnel: w314 -> [_ w318]
                  tunnel: w315 -> [_ w317]
                  frame #0 {
                  }
                  frame #1 {
                    n112 = Bundle("Y-Axis Field (kG)"=w318, "Z-Axis Field (kG)"=w317) -> (→"Cartesian Display (kG)":T6)  [unwired: 1 in]
                  }
                }
              }
              frame #1 {
                w324 = 0.1 ("y")
                n113 = Multiply(x=w322, y=w324) -> (x*y=w320:dbl)
                n114 = Multiply(x=w323, y=w324) -> (x*y=w321:dbl)
                n115 = case shown="True" w325 {
                  tunnel: w320 -> [_ w328]
                  tunnel: w321 -> [_ w327]
                  frame #0 {
                  }
                  frame #1 {
                    n116 = Bundle(w328, w327) -> (→"Cartesian Display (T)":cluster{dbl, dbl})  [unwired: 1 in]
                  }
                }
              }
            }
          }
          frame #1 {
            n117 = stacked-sequence {
              tunnel: w337 -> [w348]
              tunnel: w336 -> [w347]
              tunnel: w335 -> [w346]
              tunnel: w334 -> [w345]
              tunnel: w333 -> [w342]
              tunnel: [w340] -> w332
              tunnel: [w338] -> w330
              tunnel: [w339] -> w331
              tunnel: [w338] -> w329
              frame #0 {
                # "Field"
                n118 = call <userlib>:"Get 2D Field (Polar).vi"("Y-Axis Communications Config"=w348, "Z-Axis Communications Config"=w347, "error in"=w346) -> ("All Instruments Responded?"=w341:bool, "Radial (r) Field (kG)"=w344:dbl, "q (radians)"=w343:dbl, "error out"=w340:T5)  [unwired: 2 in]
                n119 = case shown="1" w345 {
                  tunnel: w344 -> [w350 w362]
                  tunnel: w343 -> [w352 w361]
                  tunnel: w342 -> [w351 w360]
                  tunnel: w341 -> [w353 w359]
                  tunnel: [w349 w357] -> w338
                  tunnel: [w349 w358] -> w339
                  frame #0 {
                    n120 = Multiply(x=w352, y=w351) -> (x*y=w349:dbl)
                    n121 = case shown="False" w353 {
                      tunnel: w350 -> [_ w354]
                      tunnel: w349 -> [_ w355]
                      frame #0 {
                      }
                      frame #1 {
                        n122 = Bundle(w355, "Radial (r) Field (kG)"=w354) -> (→"Polar Display (kG)":cluster{dbl, "Radial (r) Field (kG)":dbl})  [unwired: 1 in]
                      }
                    }
                  }
                  frame #1 {
                    n123 = Multiply(x=w362, y=0.1) -> (x*y=w358:dbl)
                    n124 = Multiply(x=w361, y=w360) -> (x*y=w357:dbl)
                    n125 = case shown="True" w359 {
                      tunnel: w358 -> [_ w364]
                      tunnel: w357 -> [_ w365]
                      frame #0 {
                      }
                      frame #1 {
                        n126 = Bundle(w365, w364) -> (→"Polar Display (T)":cluster{dbl, dbl})  [unwired: 1 in]
                      }
                    }
                  }
                }
              }
            }
          }
        }
      }
      frame #1 {
        # "Change PID"
        n127 = case shown="True" "Change\nPID\n(polar coordinates)" {
          tunnel: w368 -> [_ w373]
          tunnel: w367 -> [_ w372]
          frame #0 {
          }
          frame #1 {
            n128 = call "SIM960Control.vi"("New Angle"=w373, "Old angle"=w372) -> ()  [unwired: 10 in]
          }
        }
      }
    }
    n129 = local read "Ramping Control"() -> (w288:u16)
    n130 = local read "Messfile Refnum"() -> (w265:refnum<file>)
    n131 = case shown="1" w288 {
      selector: w288 -> [w375 w406 w546 w550 w565]
      tunnel: w262 -> [_ w408 _ w553 w570]
      tunnel: w261 -> [_ w407 _ w552 w569]
      tunnel: [w374 w378 w545 w551 w568] -> w287
      tunnel: [w375 w406 w546 w550 w565] -> w285
      tunnel: w284 -> [_ _ _ w549 w567]
      tunnel: w283 -> [_ _ _ _ w564]
      tunnel: w282 -> [_ _ _ _ w563]
      tunnel: w281 -> [_ w398 _ _ _]
      tunnel: w280 -> [w374 w394 w545 w547 w562]
      tunnel: w278 -> [_ w391 _ _ _]
      tunnel: w277 -> [_ w390 _ _ _]
      tunnel: w276 -> [_ w389 _ _ _]
      tunnel: w275 -> [_ w388 _ _ _]
      tunnel: w274 -> [_ w387 _ _ _]
      tunnel: w273 -> [_ w386 _ _ _]
      tunnel: w272 -> [_ w385 _ _ _]
      tunnel: w271 -> [_ w384 _ _ _]
      tunnel: w270 -> [_ w383 _ _ _]
      tunnel: w269 -> [_ w382 _ _ _]
      tunnel: w268 -> [_ w381 _ _ _]
      tunnel: w267 -> [_ w380 _ _ _]
      tunnel: w266 -> [_ w377 _ _ _]
      tunnel: w265 -> [_ w376 _ _ _]
      frame #0 {
      }
      frame #1 {
        w401 = T9."HOLDING" ("y")
        n132 = local read "Number of lines"() -> (w395:i32)
        n133 = local read "Starting index"() -> (w397:i32)
        n134 = call <userlib>:"Get Ramping Mode.vi"("Communications Config"=w408, "error in"=w394) -> ("Ramping Mode"=w404:T10, "error out"=w405:T5)  [unwired: 1 out]
        n135 = call <userlib>:"Get Ramping Mode.vi"("Communications Config"=w407, "error in"=w405) -> ("Ramping Mode"=w403:T10, "error out"=w379:T5)  [unwired: 1 out]
        n136 = Less?(x=w397, y=w395) -> (x < y?=w396:bool)
        n137 = Equal?(x=w404, y=w401) -> (x = y?=w400:bool)
        n138 = Equal?(x=w403, y=w401) -> (x = y?=w399:bool)
        n139 = Compound Arithmetic op=AND(w400, w399) -> (w402:bool)
        n140 = case shown="True" w402 {
          tunnel: w398 -> [_ w429]
          tunnel: w396 -> [_ w428]
          tunnel: "Wait between \nVectors (ms)" -> [_ w427]
          tunnel: "Wait between \nVectors" -> [_ w426]
          tunnel: w391 -> [_ w425]
          tunnel: w390 -> [_ w424]
          tunnel: w389 -> [_ w423]
          tunnel: w388 -> [_ w422]
          tunnel: w387 -> [_ w421]
          tunnel: w386 -> [_ w420]
          tunnel: w385 -> [_ w419]
          tunnel: w384 -> [_ w418]
          tunnel: w383 -> [_ w417]
          tunnel: w382 -> [_ w416]
          tunnel: w381 -> [_ w415]
          tunnel: w380 -> [_ w414]
          tunnel: w379 -> [w409 w413]
          tunnel: [w409 w412] -> w378
          tunnel: w377 -> [_ w411]
          tunnel: w376 -> [_ w410]
          frame #0 {
          }
          frame #1 {
            n141 = case shown="1" w429 {
              tunnel: w428 -> [_ w451]
              tunnel: w427 -> [_ w450]
              tunnel: w426 -> [_ w449]
              tunnel: w425 -> [_ w448]
              tunnel: w424 -> [_ w447]
              tunnel: w423 -> [_ w446]
              tunnel: w422 -> [_ w445]
              tunnel: w421 -> [_ w444]
              tunnel: w420 -> [_ w443]
              tunnel: w419 -> [_ w442]
              tunnel: w418 -> [_ w441]
              tunnel: w417 -> [_ w440]
              tunnel: w416 -> [_ w439]
              tunnel: w415 -> [_ w438]
              tunnel: w414 -> [_ w437]
              tunnel: w413 -> [w430 w436]
              tunnel: [w430 w435] -> w412
              tunnel: w411 -> [_ w434]
              tunnel: w410 -> [_ w433]
              frame #0 {
                w432 = u16 2 items=["NEXT VECTOR", "RAMPING", "HOLDING", "PAUSE", "ZERO"] ("Ramping Control")
                n142 = local write "STATUS"("Holding at current vector. Set Ramping Mode to NEXT VECTOR to continue." ("STATUS")) -> ()
                n143 = local write "Ramping Control"(w432) -> ()
              }
              frame #1 {
                # "Go to NEXT VECTOR automatically"
                n144 = case shown="True" w451 {
                  tunnel: w450 -> [_ w473]
                  tunnel: w449 -> [_ w472]
                  tunnel: w448 -> [_ w471]
                  tunnel: w447 -> [_ w470]
                  tunnel: w446 -> [_ w469]
                  tunnel: w445 -> [_ w468]
                  tunnel: w444 -> [_ w467]
                  tunnel: w443 -> [_ w466]
                  tunnel: w442 -> [_ w465]
                  tunnel: w441 -> [_ w464]
                  tunnel: w440 -> [_ w463]
                  tunnel: w439 -> [_ w462]
                  tunnel: w438 -> [_ w461]
                  tunnel: w437 -> [_ w460]
                  tunnel: w436 -> [w453 w459]
                  tunnel: [w453 w458] -> w435
                  tunnel: w434 -> [_ w457]
                  tunnel: w433 -> [_ w456]
                  frame #0 {
                    w455 = u16 2 items=["NEXT VECTOR", "RAMPING", "HOLDING", "PAUSE", "ZERO"] ("Ramping Control")
                    n145 = local write "STATUS"("Holding at current vector. Set Ramping Mode to NEXT VECTOR to continue." ("STATUS")) -> ()
                    n146 = local write "Ramping Control"(w455) -> ()
                    n147 = local write "Continue Execution?"(FALSE) -> ()
                  }
                  frame #1 {
                    n148 = stacked-sequence {
                      tunnel: w473 -> [w491 _]
                      tunnel: w472 -> [w490 _]
                      tunnel: w471 -> [w489 _]
                      tunnel: w470 -> [w488 _]
                      tunnel: w469 -> [w487 _]
                      tunnel: w468 -> [w486 _]
                      tunnel: w467 -> [w485 _]
                      tunnel: w466 -> [w484 _]
                      tunnel: w465 -> [w483 _]
                      tunnel: w464 -> [w482 _]
                      tunnel: w463 -> [w481 _]
                      tunnel: w462 -> [w480 _]
                      tunnel: w461 -> [w479 _]
                      tunnel: w460 -> [w478 _]
                      tunnel: w459 -> [w477 _]
                      tunnel: [w476 _] -> w458
                      tunnel: w457 -> [w475 _]
                      tunnel: w456 -> [w474 _]
                      frame #0 {
                        n149 = case shown="True" w490 {
                          tunnel: w491 -> [_ w509]
                          tunnel: w489 -> [_ w508]
                          tunnel: w488 -> [_ w507]
                          tunnel: w487 -> [_ w506]
                          tunnel: w486 -> [_ w505]
                          tunnel: w485 -> [_ w504]
                          tunnel: w484 -> [_ w503]
                          tunnel: w483 -> [_ w502]
                          tunnel: w482 -> [_ w501]
                          tunnel: w481 -> [_ w500]
                          tunnel: w480 -> [_ w499]
                          tunnel: w479 -> [_ w498]
                          tunnel: w478 -> [_ w497]
                          tunnel: w477 -> [w492 w496]
                          tunnel: [w492 w495] -> w476
                          tunnel: w475 -> [_ w494]
                          tunnel: w474 -> [_ w493]
                          frame #0 {
                          }
                          frame #1 {
                            n150 = stacked-sequence {
                              tunnel: w509 -> [w510 _]
                              tunnel: w508 -> [_ w542]
                              tunnel: w507 -> [_ w541]
                              tunnel: [_ w511] -> _
                              tunnel: w506 -> [_ w540]
                              tunnel: w505 -> [_ w539]
                              tunnel: w504 -> [_ w538]
                              tunnel: w503 -> [_ w537]
                              tunnel: w502 -> [_ w536]
                              tunnel: w501 -> [_ w535]
                              tunnel: w500 -> [_ w534]
                              tunnel: w499 -> [_ w533]
                              tunnel: w498 -> [_ w532]
                              tunnel: w497 -> [_ w531]
                              tunnel: w496 -> [_ w530]
                              tunnel: [_ w515] -> w495
                              tunnel: w494 -> [_ w514]
                              tunnel: w493 -> [_ w511]
                              frame #0 {
                                n151 = Wait (ms)(milliseconds to wait=w510) -> ()  [unwired: 1 out]
                              }
                              frame #1 {
                                n152 = call "ReadallDevicesv1.vi"("GPIB HP 2"=w534, "LI 3"=w538, "LI 2"=w539, "LI 1"=w540, "Nr. of Accumulations"=w514, "HP 2"=w536, "GPIB HP"=w535, "Y-Axis Field (kG)"=w542, "HP 1"=w537, "Radial (r) Field (kG) 2"=w541, "error in"=w530, "GPIB L 3"=w531, "GPIB L 2"=w532, "GPIB L 1"=w533) -> ("appended array"=w512:dbl[], "error out"=w516:errorcluster)
                                "appended array" <- w512
                                n153 = Array To Spreadsheet String(array=w512, 3:"%f" ("format string")) -> (spreadsheet string=w517:string)  [unwired: 1 in]
                                n154 = local read "measured data"() -> (w529:dbl[][])
                                n155 = Insert Into Array(array=w529, new element=w512) -> (w513:dbl[][])  [unwired: 2 in]
                                n156 = Index Array(array=w513, index (col)="X Axis") -> (element=w528:dbl[])  [unwired: 1 in]
                                n157 = Index Array(array=w513, index (col)="Y Axis") -> (element=w527:dbl[])  [unwired: 1 in]
                                n158 = Set File Position(refnum=w511, from (0:start)=1, error in=w516) -> (refnum out=w522:refnum<file>, error out=w521:errorcluster)  [unwired: 1 in]
                                n159 = Bundle("measured data"=w528, "measured data"=w527) -> (w526:T2)  [unwired: 1 in]
                                n160 = local write "measured data"(w513) -> ()
                                n161 = Write to Text File(file (use dialog)=w522, text=w517, error in=w521) -> (refnum out=w519:refnum<file>, error out=w520:errorcluster)  [unwired: 1 in, 1 out]
                                n162 = local write "XY Graph"(w526) -> ()
                                n163 = Flush File(refnum=w519, error in=w520) -> (error out=w515:errorcluster)  [unwired: 1 out]
                              }
                            }
                          }
                        }
                      }
                      frame #1 {
                        w544 = u16 0 items=["NEXT VECTOR", "RAMPING", "HOLDING", "PAUSE", "ZERO"] ("Ramping Control")
                        n164 = local write "Ramping Control"(w544) -> ()
                        n165 = local write "STATUS"("Go to NEXT VECTOR" ("STATUS")) -> ()
                      }
                    }
                  }
                }
              }
            }
          }
        }
      }
      frame #2 {
      }
      frame #3 {
        n166 = Not Equal?(x=w550, y=w549) -> (x != y?=w548:bool)
        n167 = case shown="True" w548 {
          tunnel: w553 -> [_ w561]
          tunnel: w552 -> [_ w560]
          tunnel: [w554 w558] -> w551
          tunnel: w547 -> [w554 w555]
          frame #0 {
          }
          frame #1 {
            w556 = u16 1 items=["RAMP", "PAUSE", "MANUAL UP", "MANUAL DOWN", "ZERO"] ("Ramping Mode")
            n168 = call <userlib>:"Set Ramping Mode.vi"("error in"=w555, "Ramping Mode"=w556, "Communications Config"=w561) -> ("error out"=w559:T5)
            n169 = call <userlib>:"Set Ramping Mode.vi"("error in"=w559, "Ramping Mode"=w556, "Communications Config"=w560) -> ("error out"=w558:T5)
            n170 = local write "STATUS"("All Programmers are PAUSED. Set Ramping Mode to NEXT VECTOR to continue." ("STATUS")) -> ()
          }
        }
      }
      frame #4 {
        n171 = Not Equal?(x=w565, y=w567) -> (x != y?=w566:bool)
        n172 = case shown="True" w566 {
          tunnel: w570 -> [_ w579]
          tunnel: w569 -> [_ w578]
          tunnel: [w571 w574] -> w568
          tunnel: w564 -> [_ w577]
          tunnel: w563 -> [_ w576]
          tunnel: w562 -> [w571 w572]
          frame #0 {
          }
          frame #1 {
            w573 = u16 4 items=["RAMP", "PAUSE", "MANUAL UP", "MANUAL DOWN", "ZERO"] ("Ramping Mode")
            n173 = local write "STATUS"("Zeroing vector." ("STATUS")) -> ()
            n174 = call <userlib>:"Set Ramping Mode.vi"("error in"=w572, "Ramping Mode"=w573, "Communications Config"=w579) -> ("error out"=w582:T5)
            n175 = call <userlib>:"Set Ramping Mode.vi"("error in"=w582, "Ramping Mode"=w573, "Communications Config"=w578) -> ("error out"=w575:T5)
            n176 = call <userlib>:"Set Current Ramp Rate.vi"("Communications Config"=w579, "Ramp Rate (A/sec)"=w577, "error in"=w575) -> ("error out"=w580:T5)  [unwired: 2 in]
            n177 = call <userlib>:"Set Current Ramp Rate.vi"("Communications Config"=w578, "Ramp Rate (A/sec)"=w576, "error in"=w580) -> ("error out"=w574:T5)  [unwired: 2 in]
          }
        }
      }
    }
    n178 = local read "Continue Execution?"() -> (w286:bool)
  }
  n179 = local read "Magnetic Field Units"() -> (w67:u16)
  n180 = local read "Coordinate System"() -> (w68:u16)
  n181 = while {
    tunnel: "Starting index" -> [w590]
    tunnel: w11 -> [w596]
    tunnel: w10 -> [w597]
    tunnel: w67 -> [w598]
    tunnel: w68 -> [w599]
    tunnel: w65 -> [w602]
    tunnel: "Max Ramp Rate - Y Axis (A/s)" -> [w586]
    tunnel: "Max Ramp Rate - Z Axis (A/s)" -> [w585]
    tunnel: "Magnitude Limit (kG)" -> [w587]
    tunnel: "User defined Ramp Rate (T/min)" -> [w584]
    tunnel: "User defined Ramp Rate (T/min)" -> [w583]
    i -> [w589]
    stop <- w591 continue-if-true
    n182 = local read "Field Values"() -> (w593:string[][])
    n183 = Add(x=w590, y=w589) -> (x+y=w588:i32)
    n184 = while "Wait for NEXT VECTOR setting by operator." {
      tunnel: [w606] -> w601
      tunnel: w602 -> [w606]
      stop <- w607 continue-if-true
      w605 = u16 0 items=["NEXT VECTOR", "RAMPING", "HOLDING", "PAUSE", "ZERO"] ("Ramping Control")
      n185 = local read "Ramping Control"() -> (w608:u16)
      n186 = Not Equal?(x=w605, y=w608) -> (x != y?=w607:bool)
    }
    n187 = stacked-sequence {
      tunnel: w588 -> [w610 _ w616 _]
      frame #0 {
        (unwired) -2
        n188 = Subtract(x=w610, y=2) -> (x-y=w613:i32)
        n189 = Bundle(w613, -2) -> (w611:cluster{i32, i32})  [unwired: 1 in]
        n190 = property on="Field Values" class="Tbl (strict)"("Active Cell:Active Cell"=w611) -> ()  [unwired: 2 in, 2 out]
      }
      frame #1 {
        n191 = local read "Normal color"() -> (w614:u32)
        n192 = property on="Field Values" class="Tbl (strict)"("Active Cell:Cell Background Color"=w614) -> ()  [unwired: 2 in, 2 out]
      }
      frame #2 {
        n193 = Decrement(x=w616) -> (x-1=w615:i32)
        n194 = Bundle(w615, -2) -> (w618:cluster{i32, i32})  [unwired: 1 in]
        n195 = property on="Field Values" class="Tbl (strict)"("Active Cell:Active Cell"=w618) -> ()  [unwired: 2 in, 2 out]
      }
      frame #3 {
        n196 = property on="Field Values" class="Tbl (strict)"("Active Cell:Cell Background Color"="Highlight color") -> ()  [unwired: 2 in, 2 out]
      }
    }
    n197 = Index Array(array=w593, index (row)=w588) -> (element=w600:string[])  [unwired: 1 in]
    n198 = local write "Starting index"(w588) -> ()
    n199 = Add(x=1, y=w588) -> (x+y=w603:i32)
    n200 = Number To Decimal String(number=w603) -> (decimal integer string=w592:string)  [unwired: 1 in]
    n201 = stacked-sequence {
      tunnel: [_ w644] -> w594
      tunnel: [_ w643] -> w595
      tunnel: w601 -> [_ w639]
      tunnel: w600 -> [_ w638]
      tunnel: w599 -> [_ w637]
      tunnel: w598 -> [_ w636]
      tunnel: w597 -> [_ w635]
      tunnel: w596 -> [_ w634]
      tunnel: w592 -> [_ w633]
      tunnel: w587 -> [_ w631]
      tunnel: w586 -> [_ w630]
      tunnel: w585 -> [_ w625]
      tunnel: w584 -> [_ w629]
      tunnel: w583 -> [_ w628]
      frame #0 {
        w623 = u16 1 items=["NEXT VECTOR", "RAMPING", "HOLDING", "PAUSE", "ZERO"] ("Ramping Control")
        n202 = local write "Ramping Control"(w623) -> ()
      }
      frame #1 {
        n203 = call <userlib>:"Set 2D Next Vector_entwurf.vi"("Coordinate System"=w637, "Magnetic Field Units"=w636, 3:"User defined Ramp Rate (T/min)"=w628, "Magnitude Limit (kG)"=w631, "Y-Axis Communications Config"=w635, "Input Vector"=w638, "Z-Axis Communications Config"=w634, 10:"User defined Ramp Rate (T/min)"=w629, "Max Ramp Rate - Y Axis (A/s)"=w630, "error in"=w639, "Max Ramp Rate - Z Axis (A/s)"=w625) -> ("Y-Axis Ramp Rate (T/min)"=→"Current Ramp Rate Y (T/min)":dbl, "Within Limits?"=w644:bool, "Ramp Rate along Vector (T/min)"=→"Ramp Rate along Vector (T/min)":dbl, "Z-Axis Ramp Rate (T/min)"=→"Current Ramp Rate Z (T/min)":dbl, "All Instruments Responded?"=w643:bool, "error out"=w632:T5)  [unwired: 3 in]
        n204 = Concatenate Strings("Ramping to field vector " ("STATUS"), w633, "..." ("STATUS")) -> (w640:string)
        n205 = local write "error in"(w632) -> ()
        n206 = local write "STATUS"(w640) -> ()
      }
    }
    n207 = case shown="True" w594 {
      tunnel: w595 -> [_ w621]
      frame #0 {
        n208 = local write "STATUS"("Vector magnitude limt or maximum coil current exceeded. Vector ignored. VI halted." ("STATUS")) -> ()
      }
      frame #1 {
        n209 = case shown="True" w621 {
          frame #0 {
            n210 = local write "STATUS"("Not all programmers responded. VI halted." ("STATUS")) -> ()
          }
          frame #1 {
          }
        }
      }
    }
    n211 = Compound Arithmetic op=AND(w595, w594) -> (w591:bool)
    n212 = local write "Continue Execution?"(w591) -> ()
  }
  n213 = stacked-sequence {
    tunnel: w2 -> [w656]
    tunnel: w3 -> [w657]
    tunnel: w1 -> [w647]
    tunnel: [w646] -> _
    frame #0 {
      w651 = u16 0 items=["kG", "Tesla"] ("Magnetic Field Units")
      w652 = u16 0 items=["Cartesian", "Polar"] ("Coordinate System")
      n214 = Build Array("0", "0") -> (w653:string[])
      n215 = call <userlib>:"Set 2D Next Vector_entwurf.vi"("Coordinate System"=w652, "Magnetic Field Units"=w651, "Magnitude Limit (kG)"=45.0, "Y-Axis Communications Config"=w656, "Input Vector"=w653, "Z-Axis Communications Config"=w657, "User defined Ramp Rate (T/min)"=FALSE, "Max Ramp Rate - Y Axis (A/s)"=0.05, "error in"=w647, "Max Ramp Rate - Z Axis (A/s)"=0.15) -> ("error out"=w646:T5)  [unwired: 4 in, 5 out]
    }
  }
  n216 = local read "Magnetic Field Units"() -> (w6:u16)
  n217 = local read "Coordinate System"() -> (w7:u16)
  n218 = Divide(x=180.0, y=3.141592653589793) -> (x/y=w5:dbl)
  n219 = Unbundle By Name(w11) -> ("Active Comm Interface"=w48:u16, "connection ID"=w47:refnum<k5>, "Serial Port"=w46:refnum<visa-resource-name>)
  n220 = Unbundle By Name(w10) -> ("Active Comm Interface"=w49:u16, "connection ID"=w45:refnum<k5>, "Serial Port"=w44:refnum<visa-resource-name>)
  n221 = while {
    tunnel: w5 -> [w665]
    tunnel: w6 -> [w666]
    tunnel: w3 -> [w662]
    tunnel: w2 -> [w663]
    tunnel: [w664] -> _
    tunnel: w7 -> [w664]
    tunnel: [w659] -> w4
    tunnel: w1 -> [w658]
    stop <- w660 stop-if-true
    n222 = stacked-sequence {
      seq-local: [w706 _ _] -> [_ w794 _]
      seq-local: [w705 _ _] -> [_ w791 _]
      seq-local: [w703 _ _] -> [_ w792 _]
      seq-local: [_ w778 _] -> [_ _ w848]
      tunnel: w664 -> [w711 _ w846]
      tunnel: w663 -> [w710 _ _]
      tunnel: w662 -> [w709 _ _]
      tunnel: w666 -> [w708 _ _]
      tunnel: w665 -> [w707 _ _]
      tunnel: [_ w793 _] -> w661
      tunnel: w658 -> [w704 _ _]
      tunnel: [w703 _ _] -> _
      frame #0 {
        # "Read B Field"
        n223 = case shown="0, Default" w711 {
          tunnel: w710 -> [w721 w743]
          tunnel: w709 -> [w720 w742]
          tunnel: w708 -> [w719 w741]
          tunnel: w707 -> [_ w740]
          tunnel: [w715 w739] -> w706
          tunnel: [w714 w737] -> w705
          tunnel: [w713 w738] -> w703
          tunnel: w704 -> [w712 _]
          frame #0 {
            n224 = call <userlib>:"Get 2D Field (Cartesian).vi"("Y-Axis Communications Config"=w721, "Z-Axis Communications Config"=w720, "error in"=w712) -> ("All Instruments Responded?"=w716:bool, "Y-Axis Field (kG)"=w718:dbl, "Z-Axis Field (kG)"=w717:dbl, "error out"=w715:T5)  [unwired: 2 in]
            n225 = case shown="1" w719 {
              tunnel: w718 -> [w722 w730]
              tunnel: w717 -> [w723 w731]
              tunnel: w716 -> [w724 w733]
              tunnel: [w723 w729] -> w714
              tunnel: [w722 w728] -> w713
              frame #0 {
                n226 = case shown="False" w724 {
                  tunnel: w722 -> [_ w727]
                  tunnel: w723 -> [_ w726]
                  frame #0 {
                  }
                  frame #1 {
                    n227 = Bundle("Y-Axis Field (kG)"=w727, "Z-Axis Field (kG)"=w726) -> (w725:T6)  [unwired: 1 in]
                    n228 = local write "Cartesian Display (kG)"(w725) -> ()
                  }
                }
              }
              frame #1 {
                w732 = 0.1 ("y")
                n229 = Multiply(x=w730, y=w732) -> (x*y=w728:dbl)
                n230 = Multiply(x=w731, y=w732) -> (x*y=w729:dbl)
                n231 = case shown="True" w733 {
                  tunnel: w728 -> [_ w736]
                  tunnel: w729 -> [_ w735]
                  frame #0 {
                  }
                  frame #1 {
                    n232 = Bundle(w736, w735) -> (w734:cluster{dbl, dbl})  [unwired: 1 in]
                    n233 = local write "Cartesian Display (T)"(w734) -> ()
                  }
                }
              }
            }
          }
          frame #1 {
            n234 = stacked-sequence {
              tunnel: w743 -> [w753]
              tunnel: w742 -> [w752]
              tunnel: w741 -> [w751]
              tunnel: w740 -> [w748]
              tunnel: [w746] -> w739
              tunnel: [w745] -> w737
              tunnel: [w744] -> w738
              frame #0 {
                # "Field"
                n235 = call <userlib>:"Get 2D Field (Polar).vi"("Y-Axis Communications Config"=w753, "Z-Axis Communications Config"=w752) -> ("All Instruments Responded?"=w747:bool, "Radial (r) Field (kG)"=w750:dbl, "q (radians)"=w749:dbl, "error out"=w746:T5)  [unwired: 3 in]
                n236 = case shown="1" w751 {
                  tunnel: w750 -> [w755 w767]
                  tunnel: w749 -> [w757 w766]
                  tunnel: w748 -> [w756 w765]
                  tunnel: w747 -> [w758 w764]
                  tunnel: [w755 w762] -> w745
                  tunnel: [w754 w763] -> w744
                  frame #0 {
                    n237 = Multiply(x=w757, y=w756) -> (x*y=w754:dbl)
                    n238 = case shown="True" w758 {
                      tunnel: w755 -> [_ w760]
                      tunnel: w754 -> [_ w761]
                      frame #0 {
                      }
                      frame #1 {
                        n239 = Bundle(w761, "Radial (r) Field (kG)"=w760) -> (w759:cluster{dbl, "Radial (r) Field (kG)":dbl})  [unwired: 1 in]
                        n240 = local write "Polar Display (kG)"(w759) -> ()
                      }
                    }
                  }
                  frame #1 {
                    n241 = Multiply(x=w767, y=0.1) -> (x*y=w763:dbl)
                    n242 = Multiply(x=w766, y=w765) -> (x*y=w762:dbl)
                    n243 = case shown="True" w764 {
                      tunnel: w763 -> [_ w770]
                      tunnel: w762 -> [_ w771]
                      frame #0 {
                      }
                      frame #1 {
                        n244 = Bundle(w771, w770) -> (w769:cluster{dbl, dbl})  [unwired: 1 in]
                        n245 = local write "Polar Display (T)"(w769) -> ()
                      }
                    }
                  }
                }
              }
            }
          }
        }
      }
      frame #1 {
        # "Zeile in Datei schreiben"
        # "Read and Save Devices"
        n246 = stacked-sequence {
          tunnel: [w797 _ _ _ _ _] -> w790
          tunnel: [w796 _ _ _ _ _] -> w789
          tunnel: [_ w810 _ _ _ _] -> w786
          tunnel: [_ w808 _ _ _ _] -> w785
          tunnel: [_ _ w820 _ _ _] -> w784
          tunnel: [_ _ w819 _ _ _] -> w783
          tunnel: [_ _ _ w831 _ _] -> w782
          tunnel: [_ _ _ 0.0 _ _] -> w781
          tunnel: [_ _ _ _ w837 _] -> w780
          tunnel: [_ _ _ _ _ w842] -> w779
          frame #0 {
            n247 = local read "LI 1"() -> (w795:bool)
            n248 = case shown="False" w795 {
              tunnel: ["0" ("Antwort2") w804] -> w799
              tunnel: ["0" ("Antwort1") w803] -> w798
              frame #0 {
              }
              frame #1 {
                n249 = local read "GPIB L 1"() -> (w802:string)
                n250 = call "LI-Ansteuerung.vi"("Frage2"="OUTP? 4", "Frage1"="OUTP? 1", "address string"=w802) -> ("Antwort2"=w804:string, "Antwort1"=w803:string)
              }
            }
            n251 = Fract/Exp String To Number(string=w799) -> (number=w796:dbl)  [unwired: 3 in, 1 out]
            n252 = Fract/Exp String To Number(string=w798) -> (number=w797:dbl)  [unwired: 3 in, 1 out]
          }
          frame #1 {
            n253 = local read "LI 2"() -> (w807:bool)
            n254 = case shown="False" w807 {
              tunnel: [w812 w815] -> w809
              tunnel: [w812 w814] -> w811
              frame #0 {
                w812 = "0" ("Antwort1")
              }
              frame #1 {
                n255 = local read "GPIB L 2"() -> (w813:string)
                n256 = call "LI-Ansteuerung.vi"("Frage2"="OUTP? 4", "Frage1"="OUTP? 1", "address string"=w813) -> ("Antwort2"=w815:string, "Antwort1"=w814:string)
              }
            }
            n257 = Fract/Exp String To Number(string=w809) -> (number=w808:dbl)  [unwired: 3 in, 1 out]
            n258 = Fract/Exp String To Number(string=w811) -> (number=w810:dbl)  [unwired: 3 in, 1 out]
          }
          frame #2 {
            n259 = local read "LI 3"() -> (w818:bool)
            n260 = case shown="False" w818 {
              tunnel: [w823 w826] -> w821
              tunnel: [w823 w825] -> w822
              frame #0 {
                w823 = "0" ("Antwort1")
              }
              frame #1 {
                n261 = local read "GPIB L 3"() -> (w824:string)
                n262 = call "LI-Ansteuerung.vi"("Frage2"="OUTP? 4", "Frage1"="OUTP? 1", "address string"=w824) -> ("Antwort2"=w826:string, "Antwort1"=w825:string)
              }
            }
            n263 = Fract/Exp String To Number(string=w822) -> (number=w820:dbl)  [unwired: 3 in, 1 out]
            n264 = Fract/Exp String To Number(string=w821) -> (number=w819:dbl)  [unwired: 3 in, 1 out]
          }
          frame #3 {
            n265 = local read "HP 1"() -> (w829:bool)
            n266 = case shown="True" w829 {
              tunnel: [0.0 ("Voltage") w834] -> w831
              frame #0 {
              }
              frame #1 {
                n267 = local read "GPIB HP"() -> (w833:string)
                n268 = call "HP-ReadVoltagev2.vi"("String"="meas:volt:dc? 250,0.001", "HP-Mulitmeter\nGPIB Address"=w833) -> ("Voltage"=w834:dbl)  [unwired: 9 in]
              }
            }
          }
          frame #4 {
            n269 = local read "HP 2"() -> (w836:bool)
            n270 = case shown="True" w836 {
              tunnel: [0.0 ("Voltage") w841] -> w837
              frame #0 {
              }
              frame #1 {
                n271 = local read "GPIB HP 2"() -> (w839:string)
                n272 = call "HP-ReadVoltagev2.vi"("String"="meas:volt:dc? 200,0.001", "HP-Mulitmeter\nGPIB Address"=w839) -> ("Voltage"=w841:dbl)  [unwired: 9 in]
              }
            }
          }
          frame #5 {
            n273 = Get Date/Time In Seconds() -> (seconds since 1Jan1904=w843:timestamp)
            n274 = To Double Precision Float(number=w843) -> (double precision float=w842:dbl)
          }
        }
        n275 = Build Array(w792, w791, w790, w789, w786, w785, w783, w784, w782, w781, w780, w779) -> (w778:dbl[])
        n276 = Array To Spreadsheet String(array=w778, 3:"%f" ("format string")) -> (spreadsheet string=w788:string)  [unwired: 1 in]
        n277 = local read "Messfile Refnum"() -> (w772:refnum<file>)
        n278 = Set File Position(refnum=w772, from (0:start)=1, error in=w794) -> (refnum out=w774:refnum<file>, error out=w775:errorcluster)  [unwired: 1 in]
        n279 = Write to Text File(file (use dialog)=w774, text=w788, error in=w775) -> (refnum out=w777:refnum<file>, error out=w776:errorcluster)  [unwired: 1 in, 1 out]
        n280 = Flush File(refnum=w777, error in=w776) -> (error out=w793:errorcluster)  [unwired: 1 out]
      }
      frame #2 {
        n281 = local read "X Axis"() -> (w845:enum16{"B", "phi"})
        n282 = local read "Y Axis"() -> (w844:T1)
        n283 = local read "measured data"() -> (w849:dbl[][])
        n284 = Insert Into Array(array=w849, new element=w848) -> (w847:dbl[][])  [unwired: 2 in]
        n285 = case shown="0, Default" w846 {
          tunnel: w847 -> [w865 w879]
          tunnel: w844 -> [w867 w878]
          tunnel: w845 -> [w855 w877]
          frame #0 {
            n286 = Index Array(array=w865, index (col)=1 ("disabled index (col)")) -> (element=w860:dbl[])  [unwired: 1 in]
            n287 = Index Array(array=w865, index (col)=0 ("disabled index (col)")) -> (element=w859:dbl[])  [unwired: 1 in]
            n288 = Square(x=w860) -> (x^2=w862:dbl[])
            n289 = Square(x=w859) -> (x^2=w863:dbl[])
            n290 = Index Array(array=w865, index (col)=w867) -> (element=w854:dbl[])  [unwired: 1 in]
            n291 = Divide(x=w860, y=w859) -> (x/y=w851:dbl[])
            n292 = Add(x=w863, y=w862) -> (x+y=w861:dbl[])
            n293 = Inverse Tangent(1:w851) -> (0:w850:dbl[])
            n294 = Square Root(x=w861) -> (sqrt(x)=w852:dbl[])
            n295 = Divide(x=w850, y=3.141592653589793) -> (x/y=w857:dbl[])
            n296 = Multiply(x=w857, y=180) -> (x*y=w853:dbl[])
            n297 = case shown="\"phi\"" w855 {
              tunnel: w854 -> [w870 w873]
              tunnel: w853 -> [_ w872]
              tunnel: w852 -> [w869 _]
              frame #0 {
                n298 = Bundle(w869, "measured data"=w870) -> (w868:cluster{dbl[], "measured data":dbl[]})  [unwired: 1 in]
                n299 = local write "XY Graph"(w868) -> ()
              }
              frame #1 {
                n300 = Bundle(w872, "measured data"=w873) -> (w871:cluster{dbl[], "measured data":dbl[]})  [unwired: 1 in]
                n301 = local write "XY Graph"(w871) -> ()
              }
            }
          }
          frame #1 {
            n302 = Index Array(array=w879, index (col)=w877) -> (element=w876:dbl[])  [unwired: 1 in]
            n303 = Index Array(array=w879, index (col)=w878) -> (element=w875:dbl[])  [unwired: 1 in]
            n304 = Bundle("measured data"=w876, "measured data"=w875) -> (w874:T2)  [unwired: 1 in]
            n305 = local write "XY Graph"(w874) -> ()
          }
        }
        n306 = local write "measured data"(w847) -> ()
      }
    }
    n307 = stacked-sequence {
      seq-local: [w668 _ _ _] -> [_ w678 w688 w698]
      seq-local: [w667 _ _ _] -> [_ _ w687 _]
      tunnel: w663 -> [w677 _ w690 _]
      tunnel: w662 -> [w676 _ w689 _]
      tunnel: w661 -> [w675 _ _ _]
      tunnel: [w668 _ _ _] -> w660
      tunnel: [_ _ w686 _] -> w659
      frame #0 {
        w671 = T9."HOLDING" ("y")
        n308 = call <userlib>:"Get Ramping Mode.vi"("Communications Config"=w677, "error in"=w675) -> ("Ramping Mode"=w673:T10, "error out"=w674:T5)  [unwired: 1 out]
        n309 = call <userlib>:"Get Ramping Mode.vi"("Communications Config"=w676, "error in"=w674) -> ("Ramping Mode"=w672:T10, "error out"=w667:T5)  [unwired: 1 out]
        n310 = Equal?(x=w672, y=w671) -> (x = y?=w670:bool)
        n311 = Equal?(x=w673, y=w671) -> (x = y?=w669:bool)
        n312 = And(x=w669, y=w670) -> (x .and. y?=w668:bool)
      }
      frame #1 {
        n313 = case shown="False" w678 {
          frame #0 {
          }
          frame #1 {
            n314 = flat-sequence {
              frame #0 {
                n315 = call "SIM960Poff.vi"("off/on (0/1)"="0", "Port Num- PID"="1", "GPIB-Adress"="2") -> ()  [unwired: 9 in]
              }
              frame #1 {
                n316 = call "SIM960Poff.vi"("off/on (0/1)"="0", "Port Num- PID"="3", "GPIB-Adress"="2") -> ()  [unwired: 9 in]
              }
            }
            n317 = Wait (ms)(milliseconds to wait=u32 20000) -> ()  [unwired: 1 out]
          }
        }
      }
      frame #2 {
        n318 = case shown="False" w688 {
          tunnel: w690 -> [_ w697]
          tunnel: w689 -> [_ w696]
          tunnel: [w691 w693] -> w686
          tunnel: w687 -> [w691 w692]
          frame #0 {
          }
          frame #1 {
            w694 = u16 1 items=["RAMP", "PAUSE", "MANUAL UP", "MANUAL DOWN", "ZERO"] ("Ramping Mode")
            n319 = call <userlib>:"Set Ramping Mode.vi"("error in"=w692, "Ramping Mode"=w694, "Communications Config"=w697) -> ("error out"=w695:T5)
            n320 = call <userlib>:"Set Ramping Mode.vi"("error in"=w695, "Ramping Mode"=w694, "Communications Config"=w696) -> ("error out"=w693:T5)
          }
        }
      }
      frame #3 {
        n321 = case shown="False" w698 {
          frame #0 {
          }
          frame #1 {
            n322 = call <userlib>:"430_TCP_PSoff.vi"("IP Address"="111.111.111.2", "Switch Heater Control"=FALSE) -> ()  [unwired: 5 in, 2 out]
            n323 = call <userlib>:"430_TCP_PSoff.vi"("IP Address"="111.111.111.1", "Switch Heater Control"=FALSE) -> ()  [unwired: 5 in, 2 out]
          }
        }
      }
    }
  }
  n324 = case shown="0, Default" w49 {
    tunnel: w45 -> [w882 _ _]
    tunnel: [w881 w885 w886] -> w50
    tunnel: w44 -> [_ w884 _]
    tunnel: w4 -> [w880 w883 w886]
    frame #0 {
      n325 = call <userlib>:"430_TCP_Close.vi"("error in (no error)"=w880, "connection ID"=w882) -> ("error out"=w881:errorcluster)  [unwired: 1 out]
    }
    frame #1 {
      n326 = call <userlib>:"430_RS232_Close.vi"("error in (no error)"=w883, "VISA resource name"=w884) -> ("error out"=w885:errorcluster)  [unwired: 1 in]
    }
    frame #2 {
    }
  }
  n327 = case shown="0, Default" w48 {
    tunnel: w47 -> [w889 _ _]
    tunnel: w50 -> [w888 w892 w893]
    tunnel: [w887 w891 w893] -> w43
    tunnel: w46 -> [_ w890 _]
    frame #0 {
      n328 = call <userlib>:"430_TCP_Close.vi"("error in (no error)"=w888, "connection ID"=w889) -> ("error out"=w887:errorcluster)  [unwired: 1 out]
    }
    frame #1 {
      n329 = call <userlib>:"430_RS232_Close.vi"("error in (no error)"=w892, "VISA resource name"=w890) -> ("error out"=w891:errorcluster)  [unwired: 1 in]
    }
    frame #2 {
    }
  }
  "error out" <- w43
